vi "Oxford_Data_Recorder.vi"() -> ()   [LabVIEW 2021]
uses:
  <instrlib>/Mercury iXX/Public/Controls/Comms Transport Layer.ctl
  <instrlib>/Mercury iXX/Public/Controls/Serial Settings.ctl
  <instrlib>/Mercury iXX/Public/Controls/ISOBus Address.ctl
  <instrlib>/Mercury iXX/Public/Controls/Mercury Reference.ctl
  <instrlib>/Mercury iXX/Private/Controls/Query Dynamic Reference.ctl
  <instrlib>/Stanford Research 830/Public/Data/Read (All Parameters).vi
  <instrlib>/Keithley 24XX/Public/Data/Read (Single Point).vi
  <instrlib>/Mercury iXX/Public/Libraries/System/Open/Open System.vi
  <instrlib>/Mercury iXX/Public/Libraries/System/Read/Catalogue (Read).vi
  <instrlib>/Mercury iXX/Public/Libraries/Magnet/Configuration/Read/Current to Field Factor (Read).vi
  <instrlib>/Mercury iXX/Public/Libraries/Temperature/Signals/Read/Temperature (Read).vi
  <instrlib>/Mercury iXX/Public/Libraries/Magnet/Signals/Read/Current (Read).vi
  <instrlib>/Mercury iXX/Public/Libraries/Magnet/Signals/Read/Voltage (Read).vi
  <instrlib>/Mercury iXX/Public/Libraries/Magnet/Signals/Read/Persistant Current (Read).vi
  <instrlib>/Keithley 24XX/Keithley 24XX.lvlib
  <instrlib>/Stanford Research 830/Stanford Research 830.lvlib
  <instrlib>/Mercury iXX/Mercury iXX.lvlib
  <instrlib>/Mercury iXX/Public/Libraries/System.lvlib
  <instrlib>/Mercury iXX/Public/Libraries/Magnet.lvlib
  <instrlib>/Mercury iXX/Public/Libraries/Temperature.lvlib
panel:
  in  "ISOBUS address 3":T1=-1 caption="ISOBUS address (-1)"
  in  "ISOBUS address 2":T1=-1 caption="ISOBUS address (-1)"
  in  "Mercury Reference In 2":T2
  in  "Mercury Reference In":T2
  in  "ISOBUS address":T1=-1
  in  "Mag_Ref":T2
  out "Device Details":T5
  in  "Connection Details":T7={"VISA resource name"="", "Comms Layer"=enum."Ethernet TCP/IP", "IP Address"="", "Serial Configuration"={"Baud Rate"=9600, "Parity"=0, "Data Bits"=8, "Stop Bits"=10, "Flow Control"=0}, "ISOBUS address"=-1} {"Serial Configuration"."Flow Control" items=["None", "XON/XOFF", "RTS/CTS", "XON/XOFF & RTS/CTS", "DTR/DSR", "XON/XOFF & DTR/DSR"]; "Serial Configuration"."Stop Bits" items=["1.0"=10, "2.0"=20]; "Serial Configuration"."Data Bits" items=["7"=7, "8"=8]; "Serial Configuration"."Parity" items=["None", "Odd", "Even"]; "Serial Configuration"."Baud Rate" items=["300"=300, "600"=600, "1200"=1200, "2400"=2400, "4800"=4800, "9600"=9600, "19200"=19200]}
  out "Phase-Vg":cluster{dbl[], dbl[]}[](graph)
  out "Leak-Vg":cluster{dbl[], dbl[]}[](graph)
  out "Signal-T":cluster{dbl[], dbl[]}[](graph)
  out "Signal-B":cluster{dbl[], dbl[]}[](graph)
  out "Signal-Vg":cluster{dbl[], dbl[]}[](graph)
  out "Voltage #3":sgl
  out "Leakage Current #3":sgl
  out "X-Value 3":dbl
  out "Theta-Value 3":dbl
  out "R-Value 3":dbl
  in  "Keithley #3 Ramp":bool
  in  "Keith#3 Comp. Lvl":dbl=1e-07
  in  "System #3 Enabled/Disabled":bool
  in  "Keithley #3":refnum<visa-resource-name>
  in  "SR830 #3":refnum<visa-resource-name>="GPIB0::10::INSTR"
  in  "SR830 #3 Input Connection":u16(ring) items=["Single-Ended Voltage", "Differential Voltage", "1 MOhm Current Gain", "100 MOhm Current Gain"]
  in  "SR830 #3\nInput Coupling":u16(ring) items=["AC", "DC"]
  in  "SR830 #3 Input \nShield Grounding":u16(ring) items=["Float", "Ground"]
  in  "SR830 #3 Input\nNotch Filter":u16(ring) items=["None", "Line Notch", "2x Line Notch", "Both Notch Filters"]
  in  "SR830 #3 Trigger Source":u16(ring) items=["Internal", "External"]
  in  "SR830 #3 Internal \nReference Frequency":dbl=17.0
  in  "SR830 #3 Detection Harm. Num.":dbl=1.0
  in  "SR830 #3 Sine \nOutput Amplitude":dbl=1.0
  in  "SR830 #3 Reference Source":u16(ring)=1 items=["External", "Internal"]
  in  "SR830 #3 Manual \nPhase":dbl
  in  "SR830 #3 \nAuto Phase":bool
  in  "SR830 #3 \nTime Constant":u16(ring)=9 items=["10 us", "30 us", "100 us", "300 us", "1 ms", "3 ms", "10 ms", "30 ms", "100 ms", "300 ms", "1 s", "3 s", "10 s", "30 s", "100 s", "300 s", "1 ks", "3 ks", "10 ks", "30 ks"]
  in  "SR830 #3 Low\nPass Filter Slope":u16(ring)=3 items=["6 dB/oct", "12 dB/oct", "18 db/oct", "24 dB/oct"]
  in  "SR830 #3\nSync Filter":bool
  in  "SR830 #3 \nDynamic Reserve":i16(ring)=1 items=["Auto Reserve"=-1, "High Reserve"=0, "Normal"=1, "Low Noise"=2]
  in  "SR830 #3\nSensitivity":i16(ring)=17 items=["Auto Gain"=-1, "2 nV/fA"=0, "5 nV/fA"=1, "10 nV/fA"=2, "20 nV/fA"=3, "50 nV/fA"=4, "100 nV/fA"=5, "200 nV/fA"=6, "500 nV/fA"=7, "1 uV/pA"=8, "2 uV/pA"=9, "5 uV/pA"=10, "10 uV/pA"=11, "20 uV/pA"=12, "50 uV/pA"=13, "100 uV/pA"=14, "200 uV/pA"=15, "500 uV/pA"=16, "1 mV/nA"=17, "2 mV/nA"=18, "5 mV/nA"=19, "10 mV/nA"=20, "20 mV/nA"=21, "50 mV/nA"=22, "100 mV/nA"=23, "200 mV/nA"=24, "500 mV/mA"=25, "1 V/uA"=26]
  in  "Keithley #3 Vg Init. (V)":dbl
  in  "Keithley #3 Vg Max (V)":dbl
  in  "Keithley #3 Vg Min (V)":dbl
  in  "Keithley #3 Vg Step (V)":dbl
  out "Voltage #2":sgl
  out "Leakage Current #2":sgl
  out "X-Value 2":dbl
  out "Theta-Value 2":dbl
  out "R-Value 2":dbl
  in  "Keithley #2 Ramp":bool
  in  "Keith#2 Comp. Lvl":dbl=1e-07
  in  "System #2 Enabled/Disabled":bool
  in  "Keithley #2":refnum<visa-resource-name>
  in  "SR830 #2":refnum<visa-resource-name>="GPIB0::10::INSTR"
  in  "SR830 #2 Input Connection":u16(ring) items=["Single-Ended Voltage", "Differential Voltage", "1 MOhm Current Gain", "100 MOhm Current Gain"]
  in  "SR830 #2\nInput Coupling":u16(ring) items=["AC", "DC"]
  in  "SR830 #2 Input \nShield Grounding":u16(ring) items=["Float", "Ground"]
  in  "SR830 #2 Input\nNotch Filter":u16(ring) items=["None", "Line Notch", "2x Line Notch", "Both Notch Filters"]
  in  "SR830 #2 Trigger Source":u16(ring) items=["Internal", "External"]
  in  "SR830 #2 Internal \nReference Frequency":dbl=17.0
  in  "SR830 #2 Detection Harm. Num.":dbl=1.0
  in  "SR830 #2 Sine \nOutput Amplitude":dbl=1.0
  in  "SR830 #2 Reference Source":u16(ring)=1 items=["External", "Internal"]
  in  "SR830 #2 Manual \nPhase":dbl
  in  "SR830 #2 \nAuto Phase":bool
  in  "SR830 #2 \nTime Constant":u16(ring)=9 items=["10 us", "30 us", "100 us", "300 us", "1 ms", "3 ms", "10 ms", "30 ms", "100 ms", "300 ms", "1 s", "3 s", "10 s", "30 s", "100 s", "300 s", "1 ks", "3 ks", "10 ks", "30 ks"]
  in  "SR830 #2 Low\nPass Filter Slope":u16(ring)=3 items=["6 dB/oct", "12 dB/oct", "18 db/oct", "24 dB/oct"]
  in  "SR830 #2\nSync Filter":bool
  in  "SR830 #2 \nDynamic Reserve":i16(ring)=1 items=["Auto Reserve"=-1, "High Reserve"=0, "Normal"=1, "Low Noise"=2]
  in  "SR830 #2\nSensitivity":i16(ring)=17 items=["Auto Gain"=-1, "2 nV/fA"=0, "5 nV/fA"=1, "10 nV/fA"=2, "20 nV/fA"=3, "50 nV/fA"=4, "100 nV/fA"=5, "200 nV/fA"=6, "500 nV/fA"=7, "1 uV/pA"=8, "2 uV/pA"=9, "5 uV/pA"=10, "10 uV/pA"=11, "20 uV/pA"=12, "50 uV/pA"=13, "100 uV/pA"=14, "200 uV/pA"=15, "500 uV/pA"=16, "1 mV/nA"=17, "2 mV/nA"=18, "5 mV/nA"=19, "10 mV/nA"=20, "20 mV/nA"=21, "50 mV/nA"=22, "100 mV/nA"=23, "200 mV/nA"=24, "500 mV/mA"=25, "1 V/uA"=26]
  in  "Keithley #2 Vg Init. (V)":dbl
  in  "Keithley #2 Vg Max (V)":dbl
  in  "Keithley #2 Vg Min (V)":dbl
  in  "Keithley #2 Vg Step (V)":dbl
  out "Temperature":dbl
  out "Field":dbl
  in  "Remote":bool
  out "Chamber Status":i32(ring) items=["ChamberUnknown"=0, "PurgedAndSealed"=1, "VentedAndSealed"=2, "Sealed"=3, "Purging"=4, "Venting"=5, "PreHiVac"=6, "HighVac"=7, "PumpContinuous"=8, "VentContinuous"=9, "ChamberFailure"=15]
  out "Measuring":bool
  out "R-Value":dbl
  out "Theta-Value":dbl
  out "X-Value":dbl
  out "Leakage Current #1":sgl
  out "Voltage #1":sgl
  in  "Keithley #1 Ramp":bool
  in  "Keith#1 Comp. Lvl":dbl=1e-07
  in  "Keithley #1 Vg Step (V)":dbl
  in  "Keithley #1 Vg Max (V)":dbl
  in  "Keithley #1 Vg Min (V)":dbl
  in  "Keithley #1 Vg Init. (V)":dbl
  in  "Keithley #1":refnum<visa-resource-name>
  in  "SR830 #1\nSensitivity":i16(ring)=17 items=["Auto Gain"=-1, "2 nV/fA"=0, "5 nV/fA"=1, "10 nV/fA"=2, "20 nV/fA"=3, "50 nV/fA"=4, "100 nV/fA"=5, "200 nV/fA"=6, "500 nV/fA"=7, "1 uV/pA"=8, "2 uV/pA"=9, "5 uV/pA"=10, "10 uV/pA"=11, "20 uV/pA"=12, "50 uV/pA"=13, "100 uV/pA"=14, "200 uV/pA"=15, "500 uV/pA"=16, "1 mV/nA"=17, "2 mV/nA"=18, "5 mV/nA"=19, "10 mV/nA"=20, "20 mV/nA"=21, "50 mV/nA"=22, "100 mV/nA"=23, "200 mV/nA"=24, "500 mV/mA"=25, "1 V/uA"=26]
  in  "SR830 #1 \nDynamic Reserve":i16(ring)=1 items=["Auto Reserve"=-1, "High Reserve"=0, "Normal"=1, "Low Noise"=2]
  in  "SR830 #1\nSync Filter":bool
  in  "SR830 #1 Low\nPass Filter Slope":u16(ring)=3 items=["6 dB/oct", "12 dB/oct", "18 db/oct", "24 dB/oct"]
  in  "SR830 #1 \nTime Constant":u16(ring)=8 items=["10 us", "30 us", "100 us", "300 us", "1 ms", "3 ms", "10 ms", "30 ms", "100 ms", "300 ms", "1 s", "3 s", "10 s", "30 s", "100 s", "300 s", "1 ks", "3 ks", "10 ks", "30 ks"]
  in  "SR830 #1 \nAuto Phase":bool
  in  "SR830 #1 Manual \nPhase":dbl
  in  "SR830 #1 Reference Source":u16(ring)=1 items=["External", "Internal"]
  in  "SR830 #1 Sine \nOutput Amplitude":dbl=1.0
  in  "SR830 #1 Detection Harm. Num.":dbl=1.0
  in  "SR830 #1 Internal \nReference Frequency":dbl=17.0
  in  "SR830 #1 Trigger Source":u16(ring) items=["Internal", "External"]
  in  "SR830 #1 Input\nNotch Filter":u16(ring) items=["None", "Line Notch", "2x Line Notch", "Both Notch Filters"]
  in  "SR830 #1 Input \nShield Grounding":u16(ring) items=["Float", "Ground"]
  in  "SR830 #1\nInput Coupling":u16(ring) items=["AC", "DC"]
  in  "SR830 #1 Input Connection":u16(ring) items=["Single-Ended Voltage", "Differential Voltage", "1 MOhm Current Gain", "100 MOhm Current Gain"]
  in  "SR830 #1":refnum<visa-resource-name>="GPIB0::10::INSTR"
  in  "System #1 Enabled/Disabled":bool
  in  "System Reset All?":bool
  in  "program_stop":bool
  out "Actual Save Path":path
  in  "<File Name>.txt (Don't add extension)":string
  in  "Data Save Path:":path=path "C:/Users/Nanonis Tramea/Documents/Data saving/User"
  # "Readout (Recorded)"
  # "Keithley 24XX"
  # "Ramp Settings"
  # "Current Compliance"
  # "SR830"
  # "Input Signal"
  # "Readout (Recorded)"
  # "Source / Reference"
  # "Input Filters & Sens"
  # "Readout (Recorded)"
  # "Keithley 24XX"
  # "Ramp Settings"
  # "Current Compliance"
  # "SR830"
  # "Input Signal"
  # "Readout (Recorded)"
  # "Source / Reference"
  # "Input Filters & Sens"
  # "PPMS"
  # "Readout (Recorded)"
  # "Keithley 24XX"
  # "Ramp Settings"
  # "Current Compliance"
  # "SR830"
  # "Input Signal"
  # "Readout (Recorded)"
  # "Source / Reference"
  # "Input Filters & Sens"
  # "Initialisation:\n--> Reset \n--> Instruments?"
  # "File I/O"
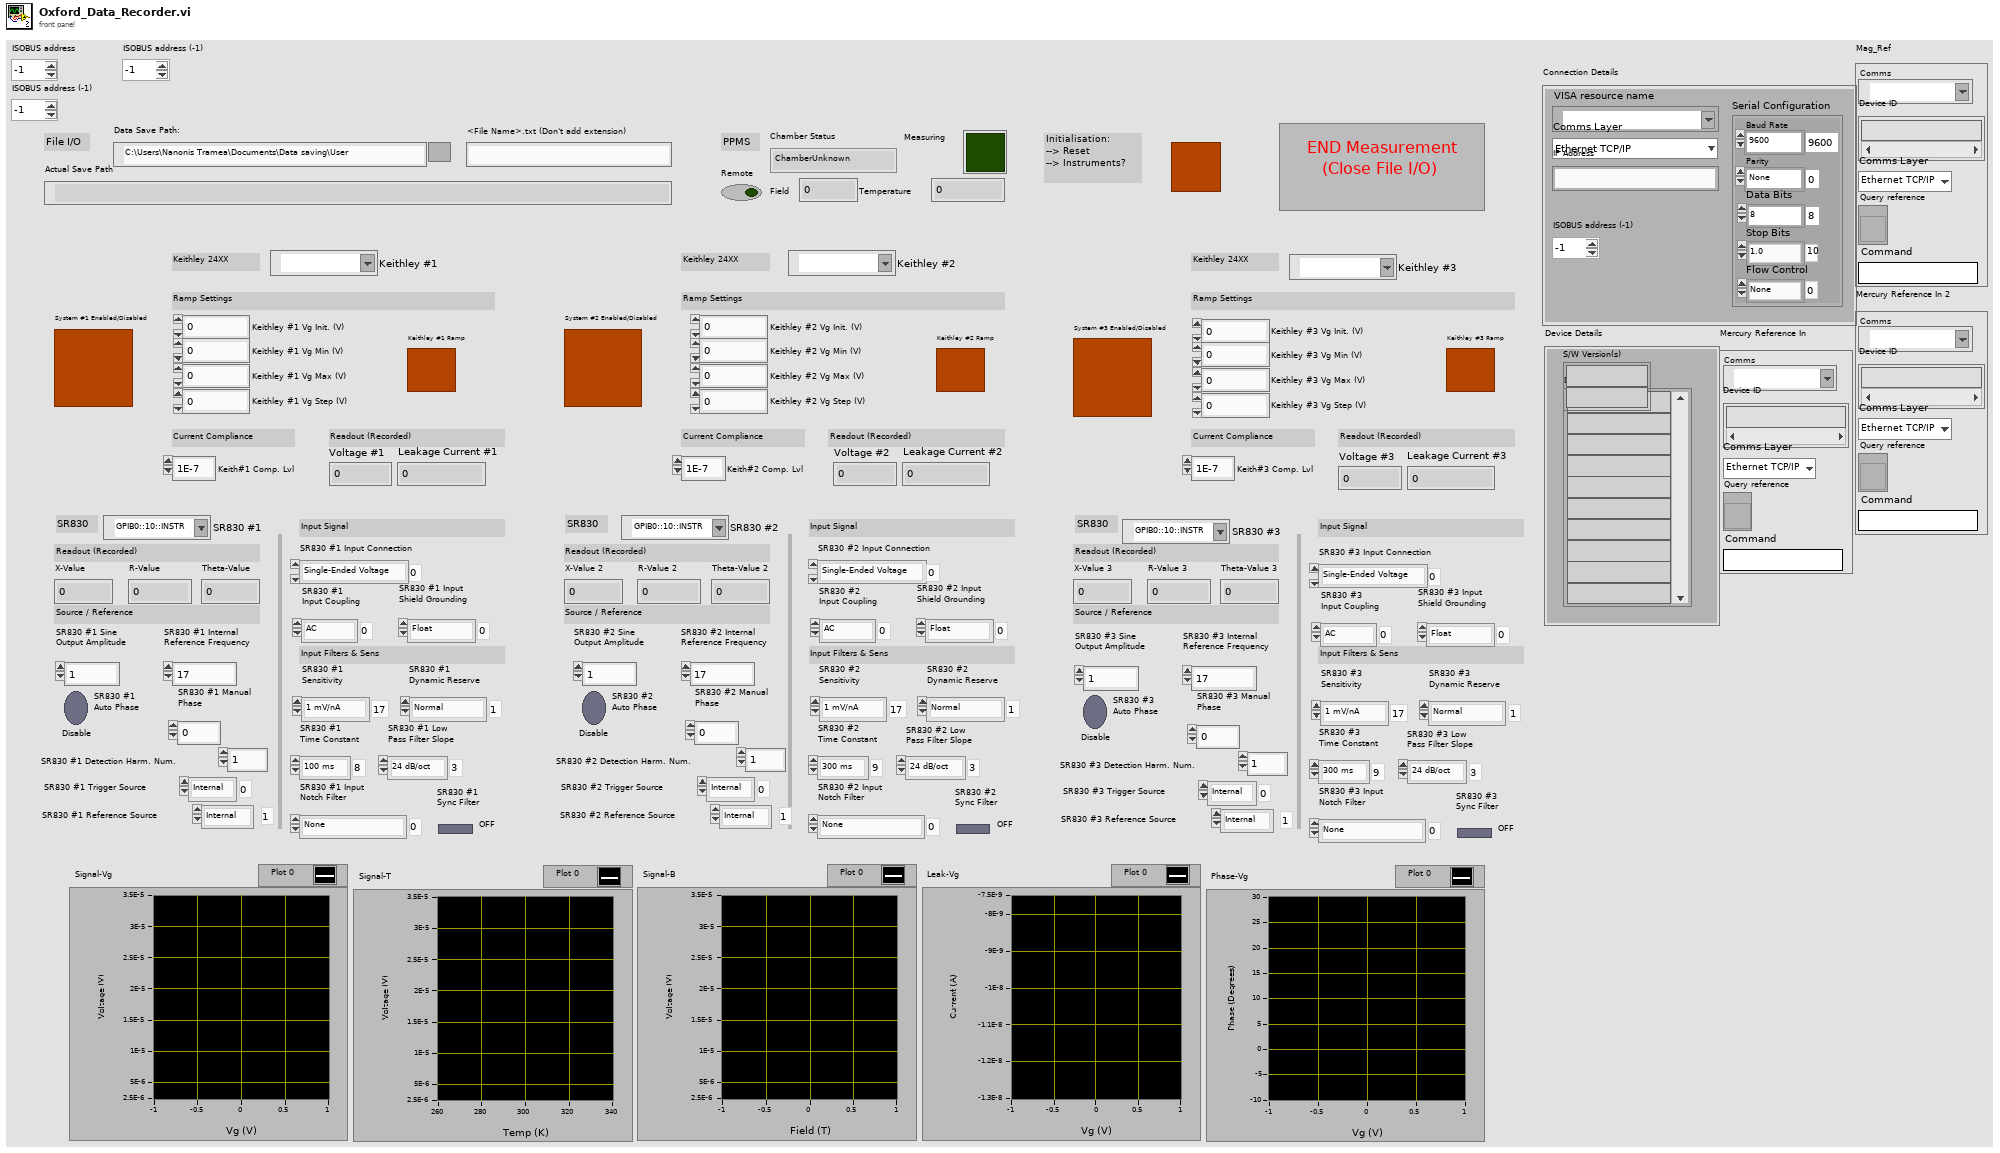
[diagram p1: front panel]
types:
  T1 = typedef "Mercury iXX.lvlib/ISOBus Address.ctl" = i32
  T2 = typedef "Mercury iXX.lvlib/Mercury Reference.ctl" = cluster{"Comms":refnum<visa-resource-name>, "Device ID":string[], "Comms Layer":T3, "Command":string, "Query reference":T4}
  T3 = typedef "Mercury iXX.lvlib/Comms Transport Layer.ctl" = enum16{"Ethernet TCP/IP", "USB", "ISOBus - RS-232", "GPIB"}
  T4 = typedef "Mercury iXX.lvlib/Query Dynamic Reference.ctl" = refnum<vi>
  T5 = cluster{"Devices":string[], "S/W Version(s)":string[]}
  T6 = typedef "Mercury iXX.lvlib/Serial Settings.ctl" = cluster{"Baud Rate":u32, "Parity":u16, "Data Bits":u16, "Stop Bits":u16, "Flow Control":u16}
  T7 = cluster{"VISA resource name":refnum<visa-resource-name>, "Comms Layer":T3, "IP Address":string, "Serial Configuration":T6, "ISOBUS address":T1}
  T8 = enum16{"open", "replace", "create", "open or create", "replace or create", "replace or create with confirmation"}
  T9 = cluster{"System #1 Enabled/Disabled":bool, "System #2 Enabled/Disabled":bool, "System #3 Enabled/Disabled":bool}
  T10 = cluster{"VISA resource name out":refnum<visa-resource-name>, "error out":errorcluster, "VISA resource name out":refnum<visa-resource-name>, "error out":errorcluster, "Keithley #1 Vg Init. (V)":dbl, "Keithley #1 Vg Max (V)":dbl, "Keithley #1 Vg Min (V)":dbl, "Keithley #1 Vg Step (V)":dbl, "Keith#1 Comp. Lvl":dbl}
  T11 = cluster{"Baud Rate":u32, "Parity":u16, "Data Bits":u16, "Stop Bits":u16, "Flow Control":u16}
  T12 = cluster{"VISA resource name out":refnum<visa-resource-name>, "error out":errorcluster, "VISA resource name out":refnum<visa-resource-name>, "error out":errorcluster, "Keithley #2 Vg Init. (V)":dbl, "Keithley #2 Vg Max (V)":dbl, "Keithley #2 Vg Min (V)":dbl, "Keithley #2 Vg Step (V)":dbl, "Keith#2 Comp. Lvl":dbl}
  T13 = cluster{"VISA resource name out":refnum<visa-resource-name>, "error out":errorcluster, "VISA resource name out":refnum<visa-resource-name>, "error out":errorcluster, "Keithley #3 Vg Init. (V)":dbl, "Keithley #3 Vg Max (V)":dbl, "Keithley #3 Vg Min (V)":dbl, "Keithley #3 Vg Step (V)":dbl, "Keith#3 Comp. Lvl":dbl}
  T14 = cluster{"array":dbl[][], "array":dbl[][], "array":dbl[][], "array":dbl[][]}
  T15 = cluster{"Voltage":sgl, "Current":sgl, "X-Value":dbl, "R-Value":dbl, "Theta-Value":dbl}
  T16 = enum8{"Enabled", "Disabled", "Disabled and Grayed Out"}
  T17 = cluster{"X-Value":dbl, "Y-Value":dbl, "R-Value":dbl, "Theta-Value":dbl, "Aux In 1 Value":dbl, "Aux In 2 Value":dbl, "Aux In 3 Value":dbl, "Aux In 4 Value":dbl, "Reference Frequency":dbl, "Channel 1 Display":dbl, "Channel 2 Display":dbl}
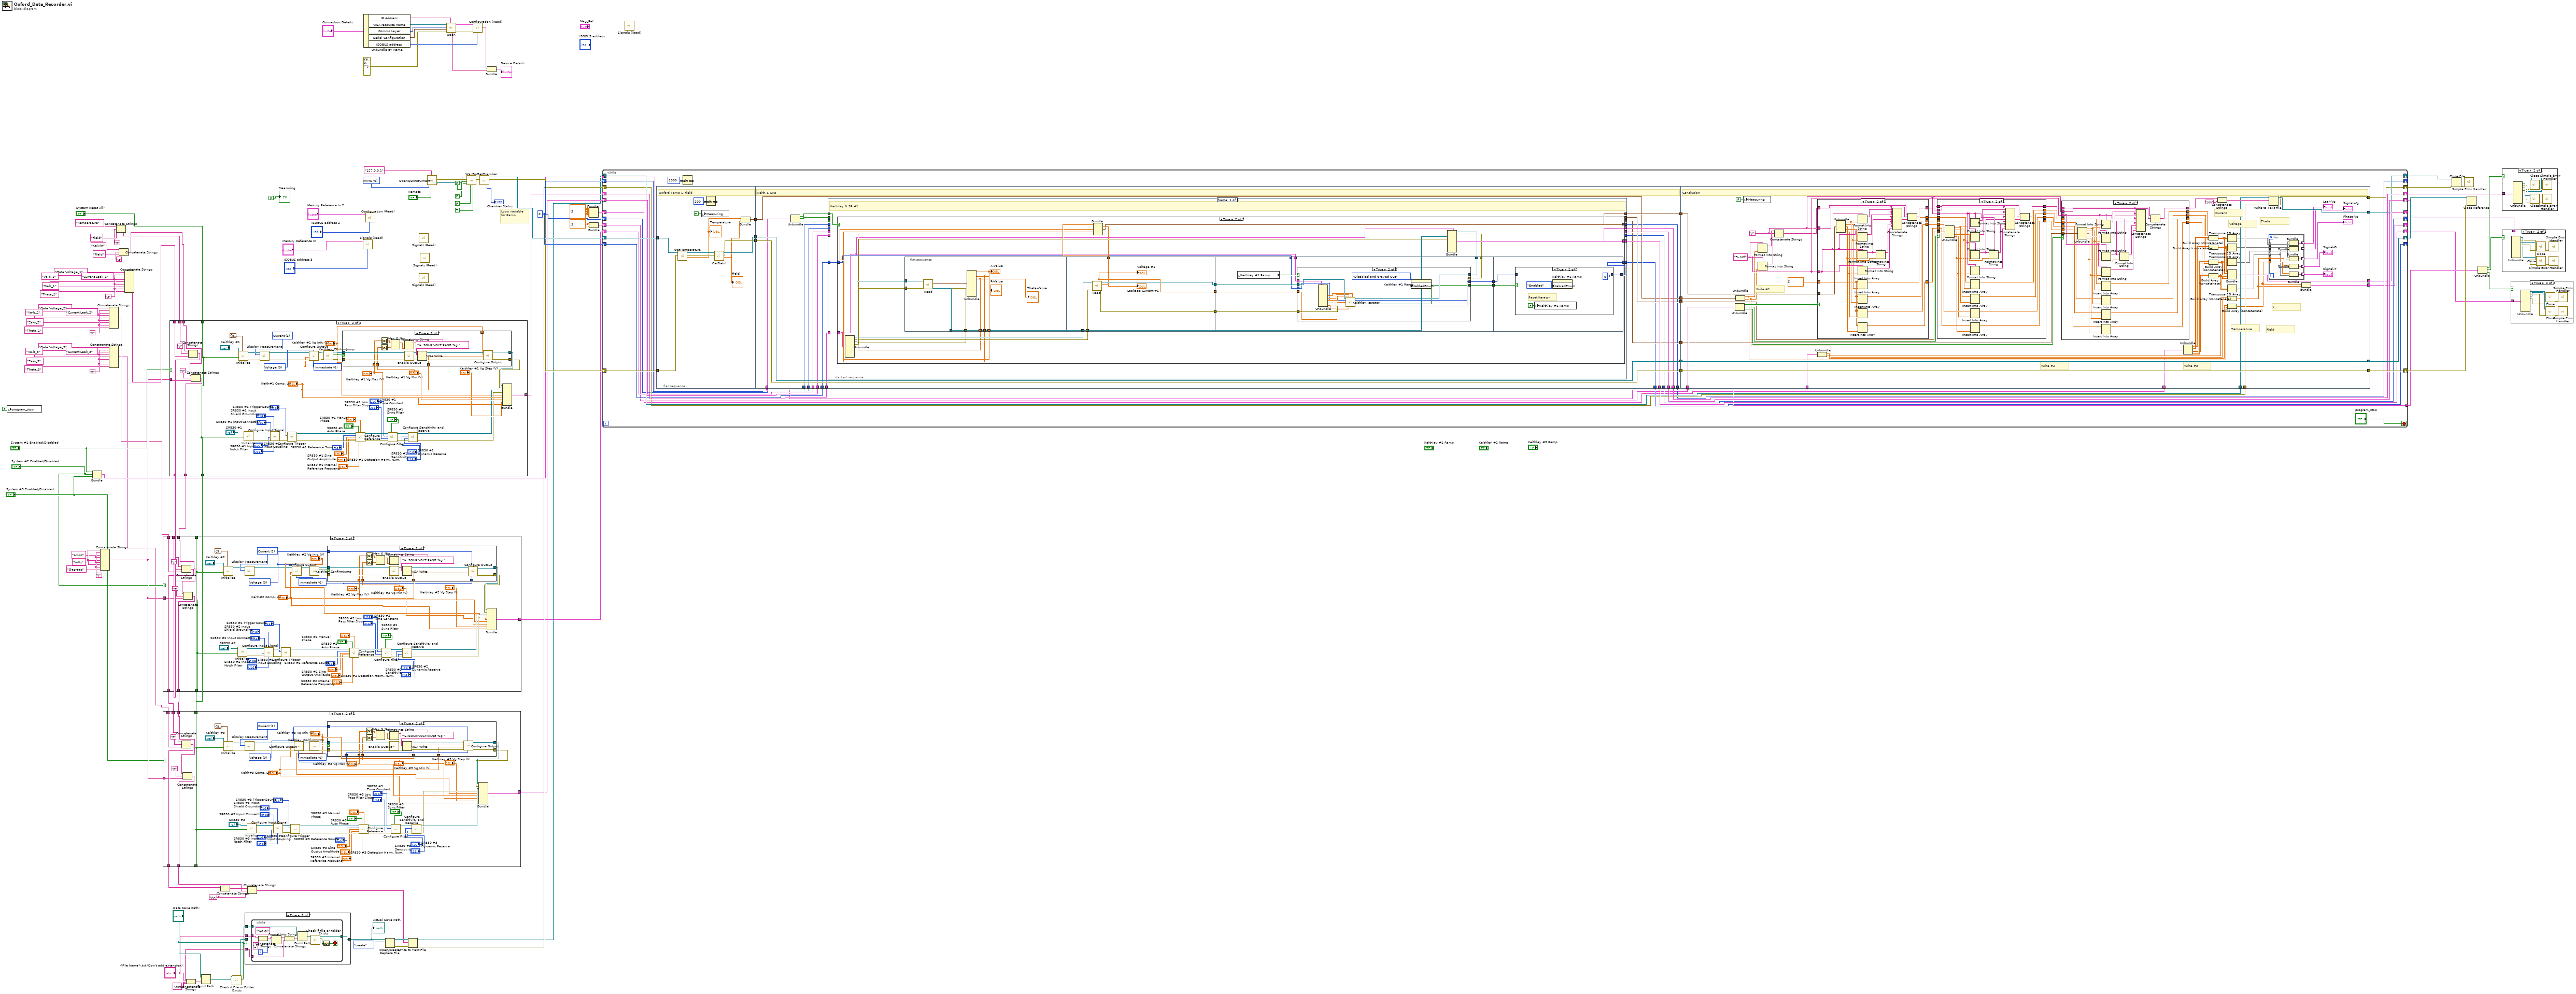
[diagram p0: block diagram]
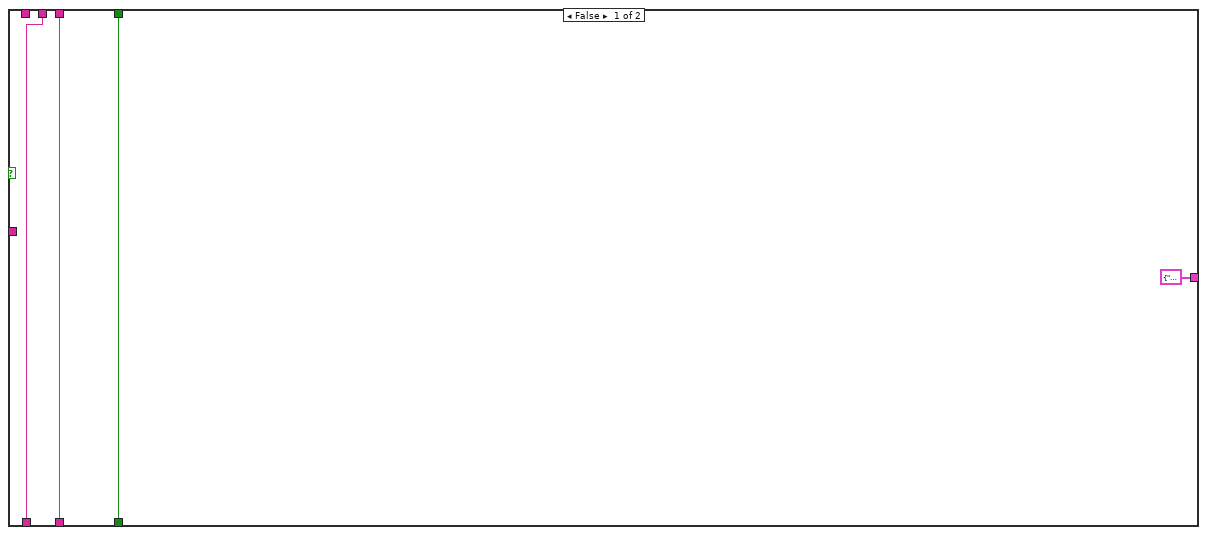
[diagram p5: hidden frame]
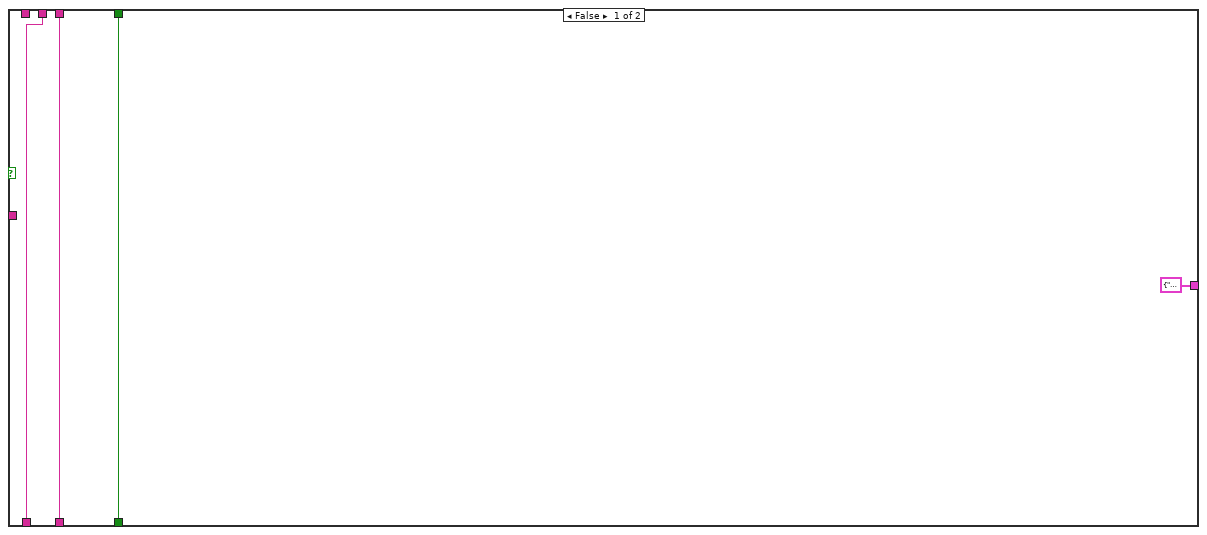
[diagram p7: hidden frame]
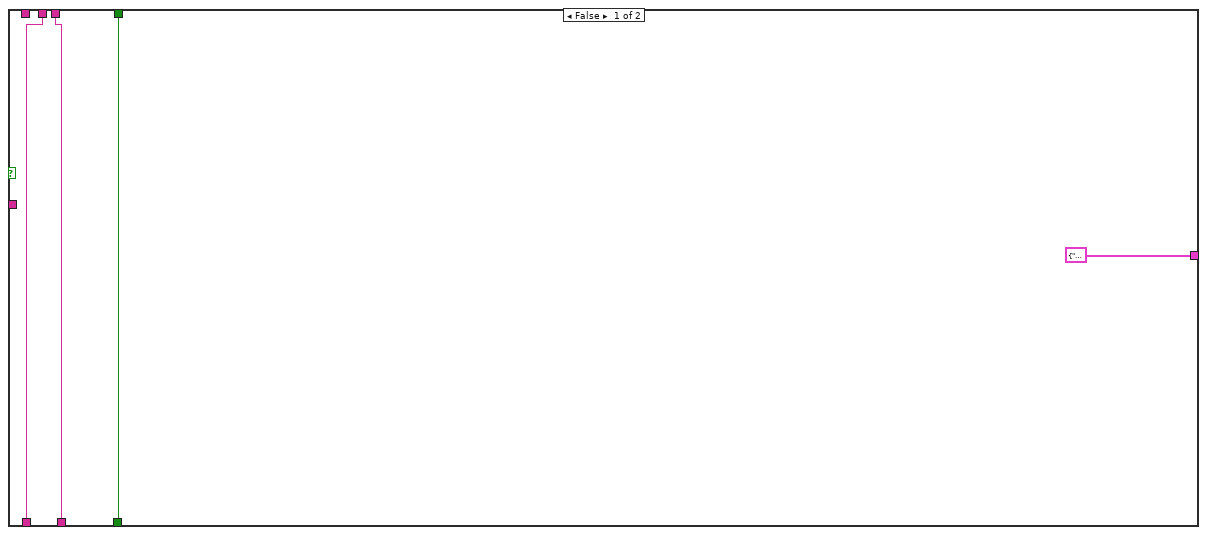
[diagram p9: hidden frame]
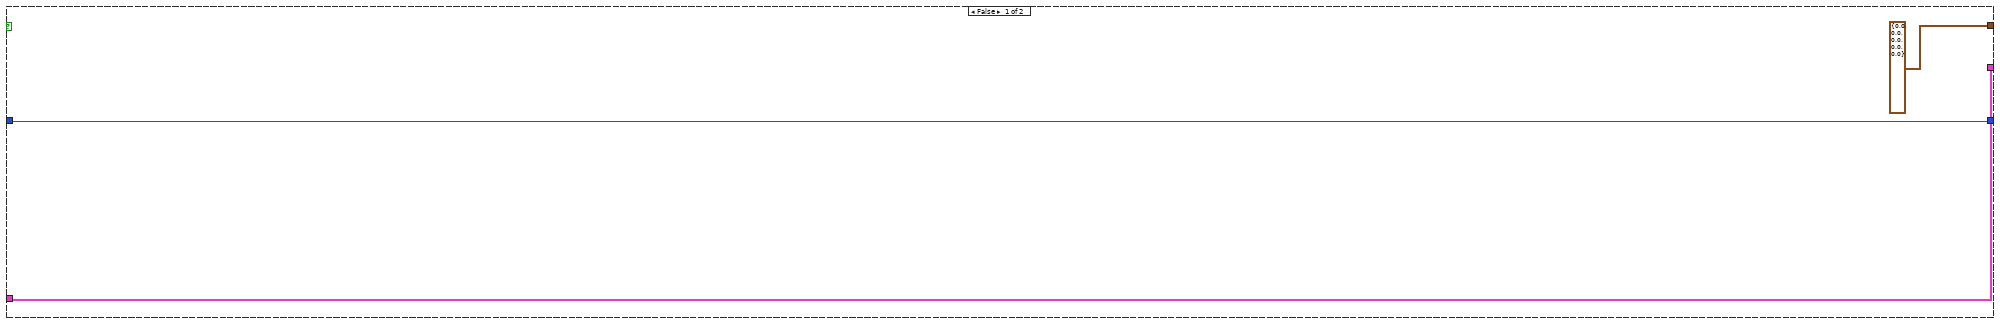
[diagram p12: hidden frame]
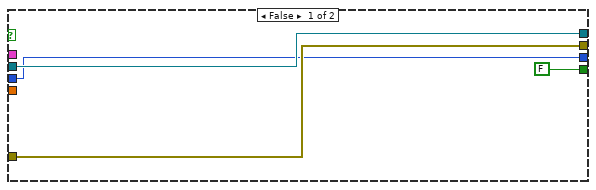
[diagram p13: hidden frame]
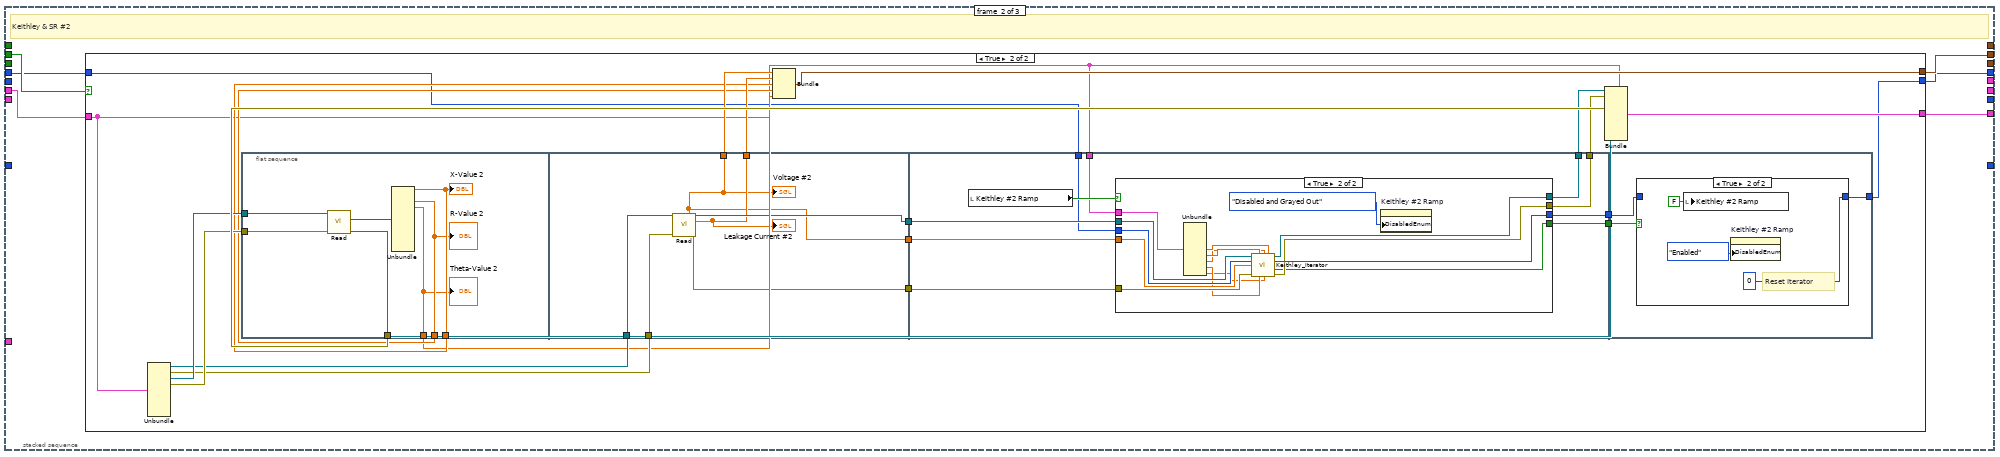
[diagram p15: hidden frame]
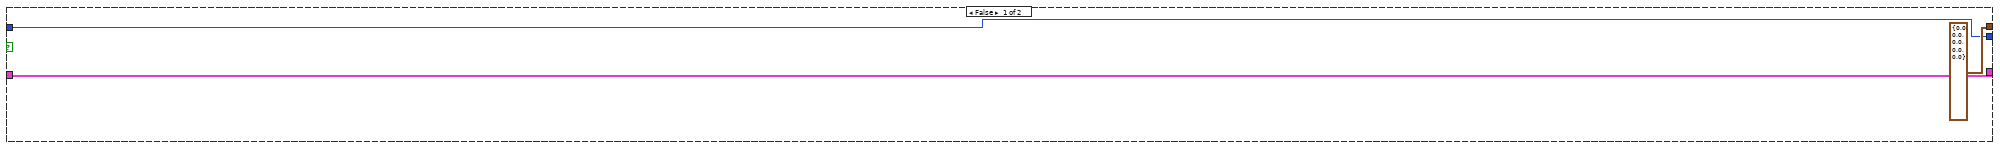
[diagram p16: hidden frame]
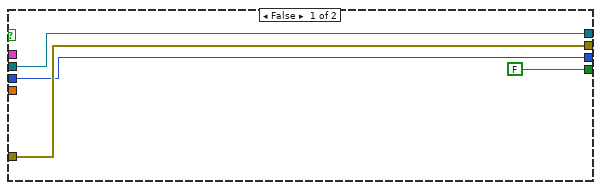
[diagram p17: hidden frame]
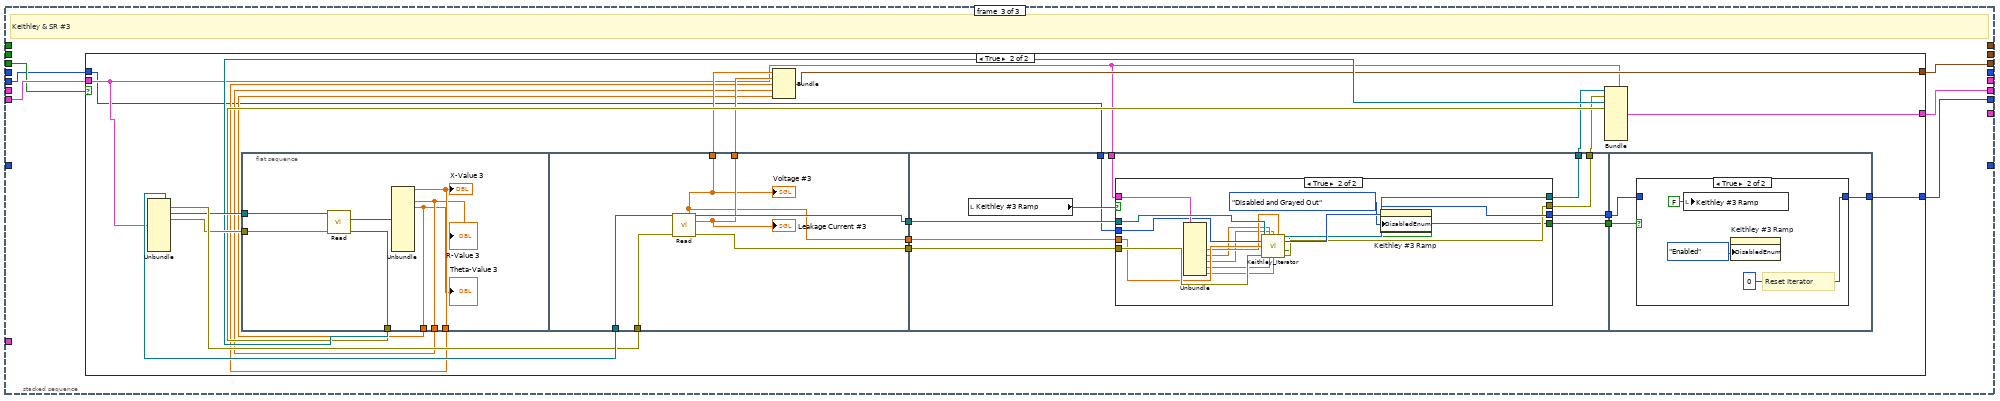
[diagram p19: hidden frame]
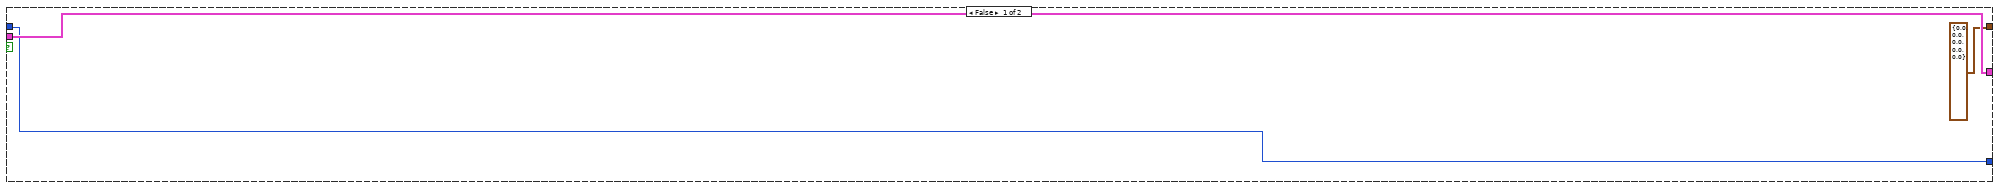
[diagram p20: hidden frame]
diagram:
  w26 = "\t"
  w32 = "\t"
  w42 = dbl[][] [] ("array")
  w44 = dbl[] [] ("array")
  w66 = 0
  w81 = "\t"
  w18 = "Volts" ("string")
  w70 = "\r\n"
  w90 = "\t"
  w95 = 0 items=["PPMS", "VersaLab", "DynaCool", "SVSM"] ("Instrument Type")
  w98 = ".txt"
  # "Loop variable \nfor Ramp"
  n1 = local write "program_stop"(FALSE ("program_stop")) -> ()
  n2 = Bundle("System #1 Enabled/Disabled"="System #1 Enabled/Disabled", "System #2 Enabled/Disabled"="System #2 Enabled/Disabled", "System #3 Enabled/Disabled"="System #3 Enabled/Disabled") -> (w51:T9)  [unwired: 1 in]
  n3 = Concatenate Strings(w18, w81, "Amps" ("string"), w81, w18, w81, w18, w81, "Degrees" ("string")) -> (w73:string)
  n4 = Concatenate Strings("Gate Voltage_2" ("string"), w32, "Current Leak_2" ("string"), w32, "Va-b_2" ("string"), w32, "Za-b_2" ("string"), w32, "Theta_2" ("string")) -> (w21:string)
  n5 = Concatenate Strings("Gate Voltage_3" ("string"), w26, "Current Leak_3" ("string"), w26, "Va-b_3" ("string"), w26, "Za-b_3" ("string"), w26, "Theta_3" ("string")) -> (w20:string)
  n6 = Concatenate Strings("Temperature" ("string"), "\t", "Field" ("string")) -> (w89:string)
  n7 = Concatenate Strings("Kelvin" ("string"), "\t", "Field" ("string")) -> (w76:string)
  n8 = Concatenate Strings("Gate Voltage_1" ("string"), w90, "Current Leak_1" ("string"), w90, "Va-b_1" ("string"), w90, "Za-b_1" ("string"), w90, "Theta_1" ("string")) -> (w84:string)
  n9 = case shown="True" "System #1 Enabled/Disabled" {
    tunnel: w84 -> [_ w179]
    tunnel: w89 -> [w119 w177]
    tunnel: [w119 w176] -> w87
    tunnel: "System Reset All?" -> [w118 w134]
    tunnel: [w118 w134] -> w86
    tunnel: w76 -> [w117 w132]
    tunnel: [w117 w131] -> w75
    tunnel: w73 -> [_ w130]
    tunnel: [T10 {"VISA resource name out"="", "error out"={"status"=FALSE, "code"=0, "source"=""}, "VISA resource name out"="", "error out"={"status"=FALSE, "code"=0, "source"=""}, "Keithley #1 Vg Init. (V)"=0.0, "Keithley #1 Vg Max (V)"=0.0, "Keithley #1 Vg Min (V)"=0.0, "Keithley #1 Vg Step (V)"=0.0, "Keith#1 Comp. Lvl"=0.0} w122] -> w57
    frame False {
    }
    frame True {
      w140 = u16 0 items=["Immediate", "Triggered"] ("Output Type  (0: Immediate)")
      w139 = u16 0 items=["Voltage", "Current"] ("Source Mode  (0: Voltage)")
      w174 = u16 1 items=["Voltage", "Current", "Resistance"] ("Displayed Measurement (0: Voltage)")
      n10 = Concatenate Strings(w177, "\t", w179) -> (w176:string)
      n11 = Concatenate Strings(w132, "\t", w130) -> (w131:string)
      n12 = call <instrlib>:"Initialize.vi"("Serial Configuration"=T11 {"Baud Rate"=9600, "Parity"=0, "Data Bits"=8, "Stop Bits"=10, "Flow Control"=0}, "Reset (True)"=w134, "VISA resource name"="Keithley #1") -> ("error out"=w172:errorcluster, "VISA resource name out"=w173:refnum<visa-resource-name>)  [unwired: 7 in]
      n13 = call <instrlib>:"Initialize.vi"("Reset (True)"=w134, "VISA resource name"="SR830 #1") -> ("error out"=w166:errorcluster, "VISA resource name out"=w167:refnum<visa-resource-name>)  [unwired: 8 in]
      n14 = call <instrlib>:"Display Measurement.vi"("error in (no error)"=w172, "Displayed Measurement (0: Voltage)"=w174, "VISA resource name"=w173) -> ("error out"=w137:errorcluster, "VISA resource name out"=w138:refnum<visa-resource-name>)  [unwired: 7 in]
      n15 = call <instrlib>:"Configure Input Signal.vi"("Input Notch Filter (0: None)"="SR830 #1 Input\nNotch Filter", "Input Shield Grounding (0: Float)"="SR830 #1 Input \nShield Grounding", "error in (no error)"=w166, "Input Coupling (0: AC)"="SR830 #1\nInput Coupling", "Input Connection (0: Single-Ended Voltage)"="SR830 #1 Input Connection", "VISA resource name"=w167) -> ("error out"=w164:errorcluster, "VISA resource name out"=w165:refnum<visa-resource-name>)  [unwired: 4 in]
      n16 = call <instrlib>:"Configure Trigger.vi"("error in (no error)"=w164, "Trigger Source (0: Internal)"="SR830 #1 Trigger Source", "VISA resource name"=w165) -> ("error out"=w162:errorcluster, "VISA resource name out"=w163:refnum<visa-resource-name>)  [unwired: 7 in]
      n17 = call <instrlib>:"Configure Output.vi"("Output Type  (0: Immediate)"=w140, "Source Mode  (0: Voltage)"=w139, "error in (no error)"=w137, "Compliance  Level (0.1)"="Keith#1 Comp. Lvl", "VISA resource name"=w138) -> ("error out"=w135:errorcluster, "VISA resource name out"=w136:refnum<visa-resource-name>)  [unwired: 5 in]
      n18 = call "Keithley_ConfirmJump.vi"("VISA resource name in"=w136, "error in"=w135, "Gate Voltage\nInitial (V)"="Keithley #1 Vg Init. (V)") -> ("VISA resource name out"=w142:refnum<visa-resource-name>, "Voltage OK?"=w143:bool, "error out"=w141:errorcluster)  [unwired: 4 in, 1 out]
      n19 = case shown="True" w143 {
        tunnel: w142 -> [w181 w191]
        tunnel: w141 -> [w180 w190]
        tunnel: [w181 w184] -> w126
        tunnel: [w180 w185] -> w125
        tunnel: "Keithley #1 Vg Max (V)" -> [_ w189]
        tunnel: "Keithley #1 Vg Min (V)" -> [_ w188]
        tunnel: "Keithley #1 Vg Init. (V)" -> [_ w183]
        tunnel: "Keith#1 Comp. Lvl" -> [_ w182]
        frame False {
        }
        frame True {
          n20 = Absolute Value(x=w189) -> (abs(x)=w193:dbl)
          n21 = Absolute Value(x=w188) -> (abs(x)=w194:dbl)
          n22 = Max & Min(x=w193, y=w194) -> (max(x,y)=w198:dbl)  [unwired: 1 out]
          n23 = Format Into String(format string="%.;SOUR:VOLT:RANG %g ", w198) -> (resulting string=w197:string)  [unwired: 2 in, 1 out]
          n24 = call <instrlib>:"Enable Output.vi"("error in (no error)"=w190, "VISA resource name"=w191) -> ("error out"=w195:errorcluster, "VISA resource name out"=w196:refnum<visa-resource-name>)  [unwired: 8 in]
          n25 = VISA Write(VISA resource name=w196, write buffer=w197, error in (no error)=w195) -> (VISA resource name out=w187:refnum<visa-resource-name>, error out=w186:errorcluster)  [unwired: 1 out]
          n26 = call <instrlib>:"Configure Output.vi"("error in (no error)"=w186, "Compliance  Level (0.1)"=w182, "Output Level (0)"=w183, "VISA resource name"=w187) -> ("error out"=w185:errorcluster, "VISA resource name out"=w184:refnum<visa-resource-name>)  [unwired: 6 in]
        }
      }
      n27 = call <instrlib>:"Configure Reference.vi"("VISA resource name"=w163, "Auto Phase (T: Enabled)"="SR830 #1 \nAuto Phase", "Manual Phase (0 Degree)"="SR830 #1 Manual \nPhase", "Reference Source (1: Internal)"="SR830 #1 Reference Source", "Sine Output Amplitude (1 V)"="SR830 #1 Sine \nOutput Amplitude", "Detection Harmonic Number (1)"="SR830 #1 Detection Harm. Num.", "error in (no error)"=w162, "Internal Reference Frequency (1000 Hz)"="SR830 #1 Internal \nReference Frequency") -> ("VISA resource name out"=w160:refnum<visa-resource-name>, "error out"=w161:errorcluster)  [unwired: 6 in]
      n28 = call <instrlib>:"Configure Filter.vi"("Enable Sync Filter (F: Disable)"="SR830 #1\nSync Filter", "error in (no error)"=w161, "Low Pass Filter Slope (1: 12dB/oct)"="SR830 #1 Low\nPass Filter Slope", "Time Constant (8: 100ms)"="SR830 #1 \nTime Constant", "VISA resource name"=w160) -> ("error out"=w146:errorcluster, "VISA resource name out"=w147:refnum<visa-resource-name>)  [unwired: 5 in]
      n29 = call <instrlib>:"Configure Sensitivity and Reserve.vi"("error in (no error)"=w146, "Sensitivity (-1: Auto gain)"="SR830 #1\nSensitivity", "Dynamic Reserve (-1: Auto Reserve)"="SR830 #1 \nDynamic Reserve", "VISA resource name"=w147) -> ("error out"=w123:errorcluster, "VISA resource name out"=w124:refnum<visa-resource-name>)  [unwired: 6 in]
      n30 = Bundle("VISA resource name out"=w126, "error out"=w125, "VISA resource name out"=w124, "error out"=w123, "Keithley #1 Vg Init. (V)"="Keithley #1 Vg Init. (V)", "Keithley #1 Vg Max (V)"="Keithley #1 Vg Max (V)", "Keithley #1 Vg Min (V)"="Keithley #1 Vg Min (V)", "Keithley #1 Vg Step (V)"="Keithley #1 Vg Step (V)", "Keith#1 Comp. Lvl"="Keith#1 Comp. Lvl") -> (w122:T10)  [unwired: 1 in]
    }
  }
  n31 = case shown="True" "System #2 Enabled/Disabled" {
    tunnel: w21 -> [_ w262]
    tunnel: w87 -> [w202 w260]
    tunnel: [w202 w259] -> w85
    tunnel: w86 -> [w201 w223]
    tunnel: [w201 w223] -> w83
    tunnel: w75 -> [w200 w221]
    tunnel: [w200 w220] -> w74
    tunnel: w73 -> [_ w219]
    tunnel: [T12 {"VISA resource name out"="", "error out"={"status"=FALSE, "code"=0, "source"=""}, "VISA resource name out"="", "error out"={"status"=FALSE, "code"=0, "source"=""}, "Keithley #2 Vg Init. (V)"=0.0, "Keithley #2 Vg Max (V)"=0.0, "Keithley #2 Vg Min (V)"=0.0, "Keithley #2 Vg Step (V)"=0.0, "Keith#2 Comp. Lvl"=0.0} w210] -> w56
    frame False {
    }
    frame True {
      w203 = u16 0 items=["Immediate", "Triggered"] ("Output Type  (0: Immediate)")
      w204 = u16 0 items=["Voltage", "Current"] ("Source Mode  (0: Voltage)")
      w257 = u16 1 items=["Voltage", "Current", "Resistance"] ("Displayed Measurement (0: Voltage)")
      n32 = Concatenate Strings(w260, "\t", w262) -> (w259:string)
      n33 = Concatenate Strings(w221, "\t", w219) -> (w220:string)
      n34 = call <instrlib>:"Initialize.vi"("Serial Configuration"=T11 {"Baud Rate"=9600, "Parity"=0, "Data Bits"=8, "Stop Bits"=10, "Flow Control"=0}, "Reset (True)"=w223, "VISA resource name"="Keithley #2") -> ("error out"=w255:errorcluster, "VISA resource name out"=w256:refnum<visa-resource-name>)  [unwired: 7 in]
      n35 = call <instrlib>:"Initialize.vi"("Reset (True)"=w223, "VISA resource name"="SR830 #2") -> ("error out"=w249:errorcluster, "VISA resource name out"=w250:refnum<visa-resource-name>)  [unwired: 8 in]
      n36 = call <instrlib>:"Display Measurement.vi"("error in (no error)"=w255, "Displayed Measurement (0: Voltage)"=w257, "VISA resource name"=w256) -> ("error out"=w208:errorcluster, "VISA resource name out"=w209:refnum<visa-resource-name>)  [unwired: 7 in]
      n37 = call <instrlib>:"Configure Input Signal.vi"("Input Notch Filter (0: None)"="SR830 #2 Input\nNotch Filter", "Input Shield Grounding (0: Float)"="SR830 #2 Input \nShield Grounding", "error in (no error)"=w249, "Input Coupling (0: AC)"="SR830 #2\nInput Coupling", "Input Connection (0: Single-Ended Voltage)"="SR830 #2 Input Connection", "VISA resource name"=w250) -> ("error out"=w247:errorcluster, "VISA resource name out"=w248:refnum<visa-resource-name>)  [unwired: 4 in]
      n38 = call <instrlib>:"Configure Trigger.vi"("error in (no error)"=w247, "Trigger Source (0: Internal)"="SR830 #2 Trigger Source", "VISA resource name"=w248) -> ("error out"=w245:errorcluster, "VISA resource name out"=w246:refnum<visa-resource-name>)  [unwired: 7 in]
      n39 = call <instrlib>:"Configure Output.vi"("Output Type  (0: Immediate)"=w203, "Source Mode  (0: Voltage)"=w204, "error in (no error)"=w208, "Compliance  Level (0.1)"="Keith#2 Comp. Lvl", "VISA resource name"=w209) -> ("error out"=w206:errorcluster, "VISA resource name out"=w205:refnum<visa-resource-name>)  [unwired: 5 in]
      n40 = call "Keithley_ConfirmJump.vi"("VISA resource name in"=w205, "error in"=w206, "Gate Voltage\nInitial (V)"="Keithley #2 Vg Init. (V)") -> ("VISA resource name out"=w225:refnum<visa-resource-name>, "Voltage OK?"=w226:bool, "error out"=w224:errorcluster)  [unwired: 4 in, 1 out]
      n41 = case shown="True" w226 {
        tunnel: w225 -> [w264 w275]
        tunnel: w224 -> [w263 w274]
        tunnel: [w264 w266] -> w218
        tunnel: [w263 w265] -> w217
        tunnel: "Keithley #2 Vg Max (V)" -> [_ w273]
        tunnel: "Keithley #2 Vg Min (V)" -> [_ w272]
        tunnel: w203 -> [_ w271]
        tunnel: w204 -> [_ w270]
        tunnel: "Keith#2 Comp. Lvl" -> [_ w269]
        frame False {
        }
        frame True {
          n42 = Absolute Value(x=w273) -> (abs(x)=w277:dbl)
          n43 = Absolute Value(x=w272) -> (abs(x)=w278:dbl)
          n44 = Max & Min(x=w277, y=w278) -> (max(x,y)=w282:dbl)  [unwired: 1 out]
          n45 = Format Into String(format string="%.;SOUR:VOLT:RANG %g ", w282) -> (resulting string=w281:string)  [unwired: 2 in, 1 out]
          n46 = call <instrlib>:"Enable Output.vi"("error in (no error)"=w274, "VISA resource name"=w275) -> ("error out"=w279:errorcluster, "VISA resource name out"=w280:refnum<visa-resource-name>)  [unwired: 8 in]
          n47 = VISA Write(VISA resource name=w280, write buffer=w281, error in (no error)=w279) -> (VISA resource name out=w268:refnum<visa-resource-name>, error out=w267:errorcluster)  [unwired: 1 out]
          n48 = call <instrlib>:"Configure Output.vi"("Output Type  (0: Immediate)"=w271, "Source Mode  (0: Voltage)"=w270, "error in (no error)"=w267, "Compliance  Level (0.1)"=w269, "VISA resource name"=w268) -> ("error out"=w265:errorcluster, "VISA resource name out"=w266:refnum<visa-resource-name>)  [unwired: 5 in]
        }
      }
      n49 = call <instrlib>:"Configure Reference.vi"("VISA resource name"=w246, "Auto Phase (T: Enabled)"="SR830 #2 \nAuto Phase", "Manual Phase (0 Degree)"="SR830 #2 Manual \nPhase", "Reference Source (1: Internal)"="SR830 #2 Reference Source", "Sine Output Amplitude (1 V)"="SR830 #2 Sine \nOutput Amplitude", "Detection Harmonic Number (1)"="SR830 #2 Detection Harm. Num.", "error in (no error)"=w245, "Internal Reference Frequency (1000 Hz)"="SR830 #2 Internal \nReference Frequency") -> ("VISA resource name out"=w243:refnum<visa-resource-name>, "error out"=w244:errorcluster)  [unwired: 6 in]
      n50 = call <instrlib>:"Configure Filter.vi"("Enable Sync Filter (F: Disable)"="SR830 #2\nSync Filter", "error in (no error)"=w244, "Low Pass Filter Slope (1: 12dB/oct)"="SR830 #2 Low\nPass Filter Slope", "Time Constant (8: 100ms)"="SR830 #2 \nTime Constant", "VISA resource name"=w243) -> ("error out"=w229:errorcluster, "VISA resource name out"=w230:refnum<visa-resource-name>)  [unwired: 5 in]
      n51 = call <instrlib>:"Configure Sensitivity and Reserve.vi"("error in (no error)"=w229, "Sensitivity (-1: Auto gain)"="SR830 #2\nSensitivity", "Dynamic Reserve (-1: Auto Reserve)"="SR830 #2 \nDynamic Reserve", "VISA resource name"=w230) -> ("error out"=w215:errorcluster, "VISA resource name out"=w216:refnum<visa-resource-name>)  [unwired: 6 in]
      n52 = Bundle("VISA resource name out"=w218, "error out"=w217, "VISA resource name out"=w216, "error out"=w215, "Keithley #2 Vg Init. (V)"="Keithley #2 Vg Init. (V)", "Keithley #2 Vg Max (V)"="Keithley #2 Vg Max (V)", "Keithley #2 Vg Min (V)"="Keithley #2 Vg Min (V)", "Keithley #2 Vg Step (V)"="Keithley #2 Vg Step (V)", "Keith#2 Comp. Lvl"="Keith#2 Comp. Lvl") -> (w210:T12)  [unwired: 1 in]
    }
  }
  n53 = case shown="True" "System #3 Enabled/Disabled" {
    tunnel: w20 -> [_ w346]
    tunnel: w85 -> [w286 w344]
    tunnel: [w286 w343] -> w82
    tunnel: w83 -> [w285 w303]
    tunnel: [w285 w303] -> _
    tunnel: w74 -> [w284 w301]
    tunnel: w73 -> [_ w300]
    tunnel: [w284 w299] -> w68
    tunnel: [T13 {"VISA resource name out"="", "error out"={"status"=FALSE, "code"=0, "source"=""}, "VISA resource name out"="", "error out"={"status"=FALSE, "code"=0, "source"=""}, "Keithley #3 Vg Init. (V)"=0.0, "Keithley #3 Vg Max (V)"=0.0, "Keithley #3 Vg Min (V)"=0.0, "Keithley #3 Vg Step (V)"=0.0, "Keith#3 Comp. Lvl"=0.0} w291] -> w55
    frame False {
    }
    frame True {
      w289 = u16 0 items=["Immediate", "Triggered"] ("Output Type  (0: Immediate)")
      w290 = u16 0 items=["Voltage", "Current"] ("Source Mode  (0: Voltage)")
      w341 = u16 1 items=["Voltage", "Current", "Resistance"] ("Displayed Measurement (0: Voltage)")
      n54 = Concatenate Strings(w344, "\t", w346) -> (w343:string)
      n55 = Concatenate Strings(w301, "\t", w300) -> (w299:string)
      n56 = call <instrlib>:"Initialize.vi"("Serial Configuration"=T11 {"Baud Rate"=9600, "Parity"=0, "Data Bits"=8, "Stop Bits"=10, "Flow Control"=0}, "Reset (True)"=w303, "VISA resource name"="Keithley #3") -> ("error out"=w339:errorcluster, "VISA resource name out"=w340:refnum<visa-resource-name>)  [unwired: 7 in]
      n57 = call <instrlib>:"Display Measurement.vi"("error in (no error)"=w339, "Displayed Measurement (0: Voltage)"=w341, "VISA resource name"=w340) -> ("error out"=w306:errorcluster, "VISA resource name out"=w307:refnum<visa-resource-name>)  [unwired: 7 in]
      n58 = call <instrlib>:"Initialize.vi"("Reset (True)"=w303, "VISA resource name"="SR830 #3") -> ("error out"=w333:errorcluster, "VISA resource name out"=w334:refnum<visa-resource-name>)  [unwired: 8 in]
      n59 = call <instrlib>:"Configure Input Signal.vi"("Input Notch Filter (0: None)"="SR830 #3 Input\nNotch Filter", "Input Shield Grounding (0: Float)"="SR830 #3 Input \nShield Grounding", "error in (no error)"=w333, "Input Coupling (0: AC)"="SR830 #3\nInput Coupling", "Input Connection (0: Single-Ended Voltage)"="SR830 #3 Input Connection", "VISA resource name"=w334) -> ("error out"=w331:errorcluster, "VISA resource name out"=w332:refnum<visa-resource-name>)  [unwired: 4 in]
      n60 = call <instrlib>:"Configure Trigger.vi"("error in (no error)"=w331, "Trigger Source (0: Internal)"="SR830 #3 Trigger Source", "VISA resource name"=w332) -> ("error out"=w329:errorcluster, "VISA resource name out"=w330:refnum<visa-resource-name>)  [unwired: 7 in]
      n61 = call <instrlib>:"Configure Output.vi"("Output Type  (0: Immediate)"=w289, "Source Mode  (0: Voltage)"=w290, "error in (no error)"=w306, "Compliance  Level (0.1)"="Keith#3 Comp. Lvl", "VISA resource name"=w307) -> ("error out"=w304:errorcluster, "VISA resource name out"=w305:refnum<visa-resource-name>)  [unwired: 5 in]
      n62 = call "Keithley_ConfirmJump.vi"("VISA resource name in"=w305, "error in"=w304, "Gate Voltage\nInitial (V)"="Keithley #3 Vg Init. (V)") -> ("VISA resource name out"=w309:refnum<visa-resource-name>, "Voltage OK?"=w310:bool, "error out"=w308:errorcluster)  [unwired: 4 in, 1 out]
      n63 = case shown="True" w310 {
        tunnel: w309 -> [w348 w360]
        tunnel: w308 -> [w347 w359]
        tunnel: [w348 w353] -> w298
        tunnel: [w347 w354] -> w297
        tunnel: "Keithley #3 Vg Max (V)" -> [_ w358]
        tunnel: "Keithley #3 Vg Min (V)" -> [_ w357]
        tunnel: w290 -> [_ w352]
        tunnel: w289 -> [_ w351]
        tunnel: "Keithley #3 Vg Init. (V)" -> [_ w350]
        tunnel: "Keith#3 Comp. Lvl" -> [_ w349]
        frame False {
        }
        frame True {
          n64 = Absolute Value(x=w358) -> (abs(x)=w362:dbl)
          n65 = Absolute Value(x=w357) -> (abs(x)=w363:dbl)
          n66 = Max & Min(x=w362, y=w363) -> (max(x,y)=w367:dbl)  [unwired: 1 out]
          n67 = Format Into String(format string="%.;SOUR:VOLT:RANG %g ", w367) -> (resulting string=w366:string)  [unwired: 2 in, 1 out]
          n68 = call <instrlib>:"Enable Output.vi"("error in (no error)"=w359, "VISA resource name"=w360) -> ("error out"=w364:errorcluster, "VISA resource name out"=w365:refnum<visa-resource-name>)  [unwired: 8 in]
          n69 = VISA Write(VISA resource name=w365, write buffer=w366, error in (no error)=w364) -> (VISA resource name out=w356:refnum<visa-resource-name>, error out=w355:errorcluster)  [unwired: 1 out]
          n70 = call <instrlib>:"Configure Output.vi"("Output Type  (0: Immediate)"=w351, "Source Mode  (0: Voltage)"=w352, "error in (no error)"=w355, "Compliance  Level (0.1)"=w349, "Output Level (0)"=w350, "VISA resource name"=w356) -> ("error out"=w354:errorcluster, "VISA resource name out"=w353:refnum<visa-resource-name>)  [unwired: 4 in]
        }
      }
      n71 = call <instrlib>:"Configure Reference.vi"("VISA resource name"=w330, "Auto Phase (T: Enabled)"="SR830 #3 \nAuto Phase", "Manual Phase (0 Degree)"="SR830 #3 Manual \nPhase", "Reference Source (1: Internal)"="SR830 #3 Reference Source", "Sine Output Amplitude (1 V)"="SR830 #3 Sine \nOutput Amplitude", "Detection Harmonic Number (1)"="SR830 #3 Detection Harm. Num.", "error in (no error)"=w329, "Internal Reference Frequency (1000 Hz)"="SR830 #3 Internal \nReference Frequency") -> ("VISA resource name out"=w327:refnum<visa-resource-name>, "error out"=w328:errorcluster)  [unwired: 6 in]
      n72 = call <instrlib>:"Configure Filter.vi"("Enable Sync Filter (F: Disable)"="SR830 #3\nSync Filter", "error in (no error)"=w328, "Low Pass Filter Slope (1: 12dB/oct)"="SR830 #3 Low\nPass Filter Slope", "Time Constant (8: 100ms)"="SR830 #3 \nTime Constant", "VISA resource name"=w327) -> ("error out"=w313:errorcluster, "VISA resource name out"=w314:refnum<visa-resource-name>)  [unwired: 5 in]
      n73 = call <instrlib>:"Configure Sensitivity and Reserve.vi"("error in (no error)"=w313, "Sensitivity (-1: Auto gain)"="SR830 #3\nSensitivity", "Dynamic Reserve (-1: Auto Reserve)"="SR830 #3 \nDynamic Reserve", "VISA resource name"=w314) -> ("error out"=w295:errorcluster, "VISA resource name out"=w296:refnum<visa-resource-name>)  [unwired: 6 in]
      n74 = Bundle("VISA resource name out"=w298, "error out"=w297, "VISA resource name out"=w296, "error out"=w295, "Keithley #3 Vg Init. (V)"="Keithley #3 Vg Init. (V)", "Keithley #3 Vg Max (V)"="Keithley #3 Vg Max (V)", "Keithley #3 Vg Min (V)"="Keithley #3 Vg Min (V)", "Keithley #3 Vg Step (V)"="Keithley #3 Vg Step (V)", "Keith#3 Comp. Lvl"="Keith#3 Comp. Lvl") -> (w291:T13)  [unwired: 1 in]
    }
  }
  n75 = Concatenate Strings("<File Name>.txt (Don't add extension)", w98) -> (w104:string)
  n76 = Build Path(base path="Data Save Path:", name or relative path=w104) -> (appended path=w103:path)
  n77 = Concatenate Strings(w82, w70) -> (w69:string)
  n78 = call <vilib>:"Check if File or Folder Exists.vi"("path"=w103) -> ("file or folder exists?"=w102:bool, "dup path"=w101:path)  [unwired: 8 in, 1 out]
  n79 = case shown="True" w102 {
    tunnel: [w368 w369] -> w96
    tunnel: w101 -> [w368 _]
    tunnel: "Data Save Path:" -> [_ w370]
    tunnel: "<File Name>.txt (Don't add extension)" -> [_ w372]
    tunnel: w98 -> [_ w371]
    frame False {
    }
    frame True {
      n80 = while {
        tunnel: w372 -> [w375]
        tunnel: w371 -> [w380]
        tunnel: w370 -> [w378]
        tunnel: [w376] -> w369
        i -> [w382]
        stop <- w384 stop-if-true
        n81 = Concatenate Strings(w375, "_" ("string")) -> (w374:string)
        n82 = Format Into String(format string="%0.0f", initial string=w374, w382) -> (resulting string=w381:string)  [unwired: 1 in, 1 out]
        n83 = Concatenate Strings(w381, w380) -> (w379:string)
        n84 = Build Path(base path=w378, name or relative path=w379) -> (appended path=w377:path)
        n85 = call <vilib>:"Check if File or Folder Exists.vi"("path"=w377) -> ("file or folder exists?"=w385:bool, "dup path"=w376:path)  [unwired: 8 in, 1 out]
        n86 = Not(x=w385) -> (.not. x?=w384:bool)
      }
    }
  }
  "Actual Save Path" <- w96
  n87 = Concatenate Strings(w69, w68, w70) -> (w67:string)
  n88 = call-poly <instrlib>:"Signals (Read).vi"("ISOBUS address"="ISOBUS address 3", "Mercury Reference In"="Mercury Reference In") -> ()  [unwired: 5 in, 5 out]
  n89 = Unbundle By Name("Connection Details") -> ("IP Address"=w11:string, "VISA resource name"=w10:refnum<visa-resource-name>, "Comms Layer"=w9:T3, "Serial Configuration"=w13:T6, "ISOBUS address"=w12:T1)
  n90 = call-poly <instrlib>:"Configuration (Read).vi"("ISOBUS address"="ISOBUS address 2", "Mercury Reference In"="Mercury Reference In 2") -> ()  [unwired: 1 in, 9 out]
  n91 = Open/Create/Replace File(file path (use dialog)=w96, operation (0:open)=T8."create") -> (refnum out=w72:refnum<file>, error out=w71:errorcluster)  [unwired: 4 in, 1 out]
  n92 = Write to Text File(file (use dialog)=w72, text=w67, error in=w71) -> (refnum out=w46:refnum<file>, error out=w62:errorcluster)  [unwired: 1 in, 1 out]
  n93 = call-poly <instrlib>:"Signals (Read).vi"() -> ()  [unwired: 3 in, 9 out]
  n94 = call-poly <instrlib>:"Signals (Read).vi"() -> ()  [unwired: 3 in, 9 out]
  n95 = call-poly <instrlib>:"Signals (Read).vi"() -> ()  [unwired: 3 in, 9 out]
  n96 = call "OpenQDInstrument.vi"("Remote"="Remote", "IP Address"="127.0.0.1", "Instrument Type"=w95) -> ("error out"=w107:errorcluster, "Instrument Ref"=w106:refnum<k24>)  [unwired: 5 in]
  n97 = call-poly <instrlib>:"Open.vi"("IP Address"=w11, "error in (no error)"=errorcluster {"status"=FALSE, "code"=0, "source"=""}, "Serial Configuration"=w13, "Comms Layer"=w9, "VISA resource name"=w10) -> ("error out"=w15:errorcluster, "Mercury Reference Out"=w16:T2, "S/W Version(s)"=w7:string[])  [unwired: 2 in, 2 out]
  n98 = call "WaitFor.vi"("Wait For Chamber"=TRUE ("WaitForChamber"), "Wait For Position"=FALSE ("WaitForPosition"), "Wait For Field"=FALSE ("WaitForField"), "Wait For Temperature"=FALSE ("WaitForTemperature"), "error in (no error)"=w107, "Instrument Ref In"=w106) -> ("error out"=w111:errorcluster, "Instrument Ref Out"=w110:refnum<k24>)  [unwired: 4 in]
  n99 = call-poly <instrlib>:"Configuration (Read).vi"("ISOBUS address"=w12, "error in"=w15, "Mercury Reference In"=w16) -> ("Devices"=w5:string[])  [unwired: 8 out]
  n100 = call "GetChamber.vi"("error in (no error)"=w111, "Instrument Ref In"=w110) -> ("Chamber\nStatus"=→"Chamber Status":i32, "error out"=w64:errorcluster, "Instrument Ref Out"=w65:refnum<k24>)  [unwired: 2 in, 1 out]
  n101 = Bundle("Devices"=w5, "S/W Version(s)"=w7) -> (→"Device Details":T5)  [unwired: 1 out]
  n102 = Bundle("array"=w42, "array"=w42, "array"=w42, "array"=w42) -> (w45:T14)  [unwired: 1 in]
  n103 = Bundle("array"=w44, "array"=w44) -> (w43:cluster{"array":dbl[], "array":dbl[]})  [unwired: 1 in]
  n104 = while {
    shift-right: [w393] -> _
    shift-left: w66 -> [w395]
    shift-right: [w392] -> _
    shift-left: w66 -> [w394]
    shift-right: [w390] -> _
    shift-left: w66 -> [w391]
    shift-right: [w416] -> w60
    shift-left: w65 -> [w419]
    shift-right: [w414] -> w61
    shift-left: w64 -> [w418]
    shift-right: [w398] -> w59
    shift-left: w46 -> [w399]
    shift-right: [w396] -> w58
    shift-left: w62 -> [w397]
    shift-right: [w408] -> w41
    shift-left: w57 -> [w411]
    shift-right: [w407] -> w39
    shift-left: w56 -> [w410]
    shift-right: [w406] -> w40
    shift-left: w55 -> [w409]
    tunnel: w51 -> [w400]
    tunnel: [w400] -> w50
    shift-right: [w386] -> _
    shift-left: w45 -> [w389]
    shift-right: [w387] -> _
    shift-left: w43 -> [w388]
    stop <- "program_stop" stop-if-true
    n105 = flat-sequence {
      tunnel: w419 -> [w428]
      tunnel: w418 -> [w427]
      tunnel: [w426] -> w417
      tunnel: [w425] -> w415
      tunnel: [w422] -> w401
      tunnel: [w454] -> w413
      tunnel: w417 -> [w454]
      tunnel: [w453] -> w412
      tunnel: w415 -> [w453]
      tunnel: w411 -> [w452]
      tunnel: w410 -> [w451]
      tunnel: w409 -> [w450]
      tunnel: [w449] -> w408
      tunnel: [w448] -> w407
      tunnel: [w447] -> w406
      tunnel: w400 -> [w446]
      tunnel: [w442] -> w405
      tunnel: [w441] -> w404
      tunnel: [w440] -> w403
      tunnel: [w439] -> w402
      tunnel: w401 -> [w439]
      tunnel: w395 -> [w438]
      tunnel: w394 -> [w437]
      tunnel: [w436] -> w393
      tunnel: [w435] -> w392
      tunnel: w391 -> [w434]
      tunnel: [w433] -> w390
      tunnel: [w764] -> w416
      tunnel: w413 -> [w764]
      tunnel: [w763] -> w414
      tunnel: w412 -> [w763]
      tunnel: w405 -> [w760]
      tunnel: w404 -> [w758]
      tunnel: w403 -> [w757]
      tunnel: w402 -> [w759]
      tunnel: w400 -> [w762]
      tunnel: w399 -> [w744]
      tunnel: w397 -> [w742]
      tunnel: [w743] -> w398
      tunnel: [w741] -> w396
      tunnel: w389 -> [w730]
      tunnel: w388 -> [w736]
      tunnel: [w735] -> w387
      tunnel: [w729] -> w386
      frame #0 {
        # "Oxford Temp & Field"
        n106 = call "GetTemperature.vi"("error in (no error)"=w427, "Instrument Ref In"=w428) -> ("Temperature"=w424:dbl, "error out"=w431:errorcluster, "Instrument Ref Out"=w432:refnum<k24>)  [unwired: 3 in, 2 out]
        "Temperature" <- w424
        n107 = local write "Measuring"(TRUE ("Measuring")) -> ()
        n108 = Wait (ms)(milliseconds to wait=u32 200) -> ()  [unwired: 1 out]
        n109 = call "GetField.vi"("error in (no error)"=w431, "Instrument Ref In"=w432) -> ("Field"=w423:dbl, "error out"=w425:errorcluster, "Instrument Ref Out"=w426:refnum<k24>)  [unwired: 3 in, 2 out]
        "Field" <- w423
        n110 = Bundle("Temperature"=w424, "Field"=w423) -> (w422:cluster{"Temperature":dbl, "Field":dbl})  [unwired: 1 in]
      }
      frame #1 {
        # "Keith & SRs"
        n111 = Unbundle(w446) -> ("System #1 Enabled/Disabled"=w445:bool, "System #2 Enabled/Disabled"=w444:bool, "System #3 Enabled/Disabled"=w443:bool)
        n112 = stacked-sequence {
          tunnel: w452 -> [w460 _ _]
          tunnel: w451 -> [_ w541 _]
          tunnel: w450 -> [_ _ w623]
          tunnel: [w459 _ _] -> w449
          tunnel: [_ w542 _] -> w448
          tunnel: [_ _ w624] -> w447
          tunnel: w445 -> [w458 _ _]
          tunnel: w444 -> [_ w540 _]
          tunnel: w443 -> [_ _ w622]
          tunnel: [w457 _ _] -> w442
          tunnel: [_ w539 _] -> w441
          tunnel: [_ _ w621] -> w440
          tunnel: w438 -> [w456 _ _]
          tunnel: w437 -> [_ w538 _]
          tunnel: [w455 _ _] -> w436
          tunnel: [_ w537 _] -> w435
          tunnel: w434 -> [_ _ w620]
          tunnel: [_ _ w619] -> w433
          frame #0 {
            # "Keithley & SR #1"
            n113 = case shown="True" w458 {
              tunnel: w460 -> [w463 w466]
              tunnel: [w463 w481] -> w459
              tunnel: [T15 {"Voltage"=0.0, "Current"=0.0, "X-Value"=0.0, "R-Value"=0.0, "Theta-Value"=0.0} w467] -> w457
              tunnel: w456 -> [w461 w465]
              tunnel: [w461 w464] -> w455
              frame False {
              }
              frame True {
                n114 = Unbundle(w466) -> ("VISA resource name out"=w478:refnum<visa-resource-name>, "error out"=w477:errorcluster, "VISA resource name out"=w480:refnum<visa-resource-name>, "error out"=w479:errorcluster)  [unwired: 5 out]
                n115 = flat-sequence {
                  tunnel: [w494] -> w474
                  tunnel: [w493] -> w473
                  tunnel: [w491] -> w470
                  tunnel: [w490] -> w469
                  tunnel: [w489] -> w468
                  tunnel: w480 -> [w488]
                  tunnel: w479 -> [w487]
                  tunnel: [w500] -> w486
                  tunnel: [w499] -> w485
                  tunnel: [w495] -> w484
                  tunnel: [w498] -> w471
                  tunnel: w478 -> [w497]
                  tunnel: w477 -> [w496]
                  tunnel: [w495] -> w472
                  tunnel: w486 -> [w509]
                  tunnel: w485 -> [w508]
                  tunnel: [w507] -> w475
                  tunnel: w484 -> [w506]
                  tunnel: [w510] -> w483
                  tunnel: [w505] -> w482
                  tunnel: [w504] -> w476
                  tunnel: w466 -> [w502]
                  tunnel: w465 -> [w501]
                  tunnel: [w531] -> w464
                  tunnel: w483 -> [w532]
                  tunnel: w482 -> [w530]
                  frame #0 {
                    n116 = call-poly <instrlib>:"Read.vi"("error in (no error)"=w487, "VISA resource name"=w488) -> ("error out"=w493:errorcluster, "Parameter Values"=w492:T17, "VISA resource name out"=w494:refnum<visa-resource-name>)  [unwired: 7 in]
                    n117 = Unbundle(w492) -> ("X-Value"=w491:dbl, "R-Value"=w490:dbl, "Theta-Value"=w489:dbl)  [unwired: 8 out]
                    "X-Value" <- w491
                    "Theta-Value" <- w489
                    "R-Value" <- w490
                  }
                  frame #1 {
                    n118 = call-poly <instrlib>:"Read.vi"("VISA resource name"=w497, "error in (no error)"=w496) -> ("Voltage"=w495:sgl, "VISA resource name out"=w500:refnum<visa-resource-name>, "Current"=w498:sgl, "error out"=w499:errorcluster)  [unwired: 7 in, 3 out]
                    "Voltage #1" <- w495
                    "Leakage Current #1" <- w498
                  }
                  frame #2 {
                    n119 = local read "Keithley #1 Ramp"() -> (w503:bool)
                    n120 = case shown="True" w503 {
                      tunnel: [w512 w529] -> w510
                      tunnel: w509 -> [w514 w528]
                      tunnel: w508 -> [w513 w527]
                      tunnel: [w513 w526] -> w507
                      tunnel: [w514 w525] -> w504
                      tunnel: w506 -> [_ w524]
                      tunnel: [FALSE ("END?") w523] -> w505
                      tunnel: w502 -> [_ w521]
                      tunnel: w501 -> [w512 w515]
                      frame False {
                      }
                      frame True {
                        n121 = Unbundle(w521) -> ("Keithley #1 Vg Init. (V)"=w520:dbl, "Keithley #1 Vg Max (V)"=w519:dbl, "Keithley #1 Vg Min (V)"=w518:dbl, "Keithley #1 Vg Step (V)"=w517:dbl, "Keith#1 Comp. Lvl"=w516:dbl)  [unwired: 4 out]
                        n122 = call "Keithley_Iterator.vi"("VISA resource name"=w528, "High Voltage"=w519, "Low Voltage"=w518, "Initial Voltage"=w520, "Iteration Input"=w515, "Current Voltage"=w524, "error in (no error)"=w527, "Voltage Step"=w517, "Compliance  Level (0.1)"=w516) -> ("VISA resource name out"=w525:refnum<visa-resource-name>, "Iteration Output"=w529:i32, "END?"=w523:bool, "error out"=w526:errorcluster)  [unwired: 2 in, 1 out]
                        n123 = property on="Keithley #1 Ramp" class="Bool (strict)"("DisabledEnum"=T16."Disabled and Grayed Out" ("Disabled")) -> ()  [unwired: 2 in, 2 out]
                      }
                    }
                  }
                  frame #3 {
                    n124 = case shown="True" w530 {
                      tunnel: w532 -> [w533 _]
                      tunnel: [w533 0 ("Iteration Output")] -> w531
                      frame False {
                      }
                      frame True {
                        # "Reset Iterator"
                        n125 = local write "Keithley #1 Ramp"(FALSE ("Keithley #1 Ramp")) -> ()
                        n126 = property on="Keithley #1 Ramp" class="Bool (strict)"("DisabledEnum"=T16."Enabled" ("Disabled")) -> ()  [unwired: 2 in, 2 out]
                      }
                    }
                  }
                }
                n127 = Bundle("Voltage"=w472, "Current"=w471, "X-Value"=w470, "R-Value"=w469, "Theta-Value"=w468) -> (w467:T15)  [unwired: 1 in]
                n128 = Bundle(cluster=w466, "VISA resource name out"=w476, "error out"=w475, "VISA resource name out"=w474, "error out"=w473) -> (w481:T10)  [unwired: 5 in]
              }
            }
          }
          frame #1 {
            # "Keithley & SR #2"
            n129 = case shown="True" w540 {
              tunnel: [w545 w563] -> w542
              tunnel: w541 -> [w545 w547]
              tunnel: [T15 {"Voltage"=0.0, "Current"=0.0, "X-Value"=0.0, "R-Value"=0.0, "Theta-Value"=0.0} w549] -> w539
              tunnel: w538 -> [w543 w548]
              tunnel: [w543 w546] -> w537
              frame False {
              }
              frame True {
                n130 = Unbundle(w547) -> ("VISA resource name out"=w556:refnum<visa-resource-name>, "error out"=w555:errorcluster, "VISA resource name out"=w558:refnum<visa-resource-name>, "error out"=w557:errorcluster)  [unwired: 5 out]
                n131 = flat-sequence {
                  tunnel: [w576] -> w562
                  tunnel: [w575] -> w561
                  tunnel: [w573] -> w552
                  tunnel: [w572] -> w551
                  tunnel: [w571] -> w550
                  tunnel: w558 -> [w570]
                  tunnel: w557 -> [w569]
                  tunnel: [w582] -> w568
                  tunnel: [w581] -> w567
                  tunnel: [w579] -> w566
                  tunnel: [w580] -> w553
                  tunnel: [w579] -> w554
                  tunnel: w556 -> [w578]
                  tunnel: w555 -> [w577]
                  tunnel: w568 -> [w591]
                  tunnel: w567 -> [w590]
                  tunnel: [w589] -> w559
                  tunnel: [w588] -> w560
                  tunnel: w566 -> [w587]
                  tunnel: [w592] -> w565
                  tunnel: [w586] -> w564
                  tunnel: w548 -> [w584]
                  tunnel: w547 -> [w583]
                  tunnel: [w613] -> w546
                  tunnel: w565 -> [w614]
                  tunnel: w564 -> [w612]
                  frame #0 {
                    n132 = call-poly <instrlib>:"Read.vi"("error in (no error)"=w569, "VISA resource name"=w570) -> ("error out"=w575:errorcluster, "Parameter Values"=w574:T17, "VISA resource name out"=w576:refnum<visa-resource-name>)  [unwired: 7 in]
                    n133 = Unbundle(w574) -> ("X-Value"=w573:dbl, "R-Value"=w572:dbl, "Theta-Value"=w571:dbl)  [unwired: 8 out]
                    "X-Value 2" <- w573
                    "Theta-Value 2" <- w571
                    "R-Value 2" <- w572
                  }
                  frame #1 {
                    n134 = call-poly <instrlib>:"Read.vi"("VISA resource name"=w578, "error in (no error)"=w577) -> ("Voltage"=w579:sgl, "VISA resource name out"=w582:refnum<visa-resource-name>, "Current"=w580:sgl, "error out"=w581:errorcluster)  [unwired: 7 in, 3 out]
                    "Voltage #2" <- w579
                    "Leakage Current #2" <- w580
                  }
                  frame #2 {
                    n135 = local read "Keithley #2 Ramp"() -> (w585:bool)
                    n136 = case shown="True" w585 {
                      tunnel: [w594 w611] -> w592
                      tunnel: w591 -> [w596 w610]
                      tunnel: w590 -> [w595 w609]
                      tunnel: [w595 w608] -> w589
                      tunnel: [w596 w607] -> w588
                      tunnel: w587 -> [_ w606]
                      tunnel: [FALSE ("END?") w605] -> w586
                      tunnel: w584 -> [w594 w603]
                      tunnel: w583 -> [_ w602]
                      frame False {
                      }
                      frame True {
                        n137 = Unbundle(w602) -> ("Keithley #2 Vg Init. (V)"=w601:dbl, "Keithley #2 Vg Max (V)"=w600:dbl, "Keithley #2 Vg Min (V)"=w599:dbl, "Keithley #2 Vg Step (V)"=w598:dbl, "Keith#2 Comp. Lvl"=w597:dbl)  [unwired: 4 out]
                        n138 = call "Keithley_Iterator.vi"("VISA resource name"=w610, "High Voltage"=w600, "Low Voltage"=w599, "Initial Voltage"=w601, "Iteration Input"=w603, "Current Voltage"=w606, "error in (no error)"=w609, "Voltage Step"=w598, "Compliance  Level (0.1)"=w597) -> ("VISA resource name out"=w607:refnum<visa-resource-name>, "Iteration Output"=w611:i32, "END?"=w605:bool, "error out"=w608:errorcluster)  [unwired: 2 in, 1 out]
                        n139 = property on="Keithley #2 Ramp" class="Bool (strict)"("DisabledEnum"=T16."Disabled and Grayed Out" ("Disabled")) -> ()  [unwired: 2 in, 2 out]
                      }
                    }
                  }
                  frame #3 {
                    n140 = case shown="True" w612 {
                      tunnel: w614 -> [w615 _]
                      tunnel: [w615 0 ("Iteration Output")] -> w613
                      frame False {
                      }
                      frame True {
                        # "Reset Iterator"
                        n141 = local write "Keithley #2 Ramp"(FALSE ("Keithley #1 Ramp")) -> ()
                        n142 = property on="Keithley #2 Ramp" class="Bool (strict)"("DisabledEnum"=T16."Enabled" ("Disabled")) -> ()  [unwired: 2 in, 2 out]
                      }
                    }
                  }
                }
                n143 = Bundle("Voltage"=w554, "Current"=w553, "X-Value"=w552, "R-Value"=w551, "Theta-Value"=w550) -> (w549:T15)  [unwired: 1 in]
                n144 = Bundle(cluster=w547, "VISA resource name out"=w560, "error out"=w559, "VISA resource name out"=w562, "error out"=w561) -> (w563:T12)  [unwired: 5 in]
              }
            }
          }
          frame #2 {
            # "Keithley & SR #3"
            n145 = case shown="True" w622 {
              tunnel: [w627 w645] -> w624
              tunnel: w623 -> [w627 w630]
              tunnel: [T15 {"Voltage"=0.0, "Current"=0.0, "X-Value"=0.0, "R-Value"=0.0, "Theta-Value"=0.0} w631] -> w621
              tunnel: w620 -> [w625 w629]
              tunnel: [w625 w628] -> w619
              frame False {
              }
              frame True {
                n146 = Unbundle(w630) -> ("VISA resource name out"=w644:refnum<visa-resource-name>, "error out"=w643:errorcluster, "VISA resource name out"=w642:refnum<visa-resource-name>, "error out"=w641:errorcluster)  [unwired: 5 out]
                n147 = flat-sequence {
                  tunnel: [w658] -> w640
                  tunnel: [w657] -> w639
                  tunnel: [w655] -> w634
                  tunnel: [w654] -> w633
                  tunnel: [w653] -> w632
                  tunnel: w642 -> [w652]
                  tunnel: w641 -> [w651]
                  tunnel: [w664] -> w650
                  tunnel: [w663] -> w649
                  tunnel: [w661] -> w648
                  tunnel: [w662] -> w635
                  tunnel: [w661] -> w636
                  tunnel: w644 -> [w660]
                  tunnel: w643 -> [w659]
                  tunnel: w650 -> [w673]
                  tunnel: w649 -> [w672]
                  tunnel: [w671] -> w637
                  tunnel: [w670] -> w638
                  tunnel: w648 -> [w669]
                  tunnel: [w674] -> w647
                  tunnel: [w668] -> w646
                  tunnel: w630 -> [w666]
                  tunnel: w629 -> [w665]
                  tunnel: [w695] -> w628
                  tunnel: w647 -> [w696]
                  tunnel: w646 -> [w694]
                  frame #0 {
                    n148 = call-poly <instrlib>:"Read.vi"("error in (no error)"=w651, "VISA resource name"=w652) -> ("error out"=w657:errorcluster, "Parameter Values"=w656:T17, "VISA resource name out"=w658:refnum<visa-resource-name>)  [unwired: 7 in]
                    n149 = Unbundle(w656) -> ("X-Value"=w655:dbl, "R-Value"=w654:dbl, "Theta-Value"=w653:dbl)  [unwired: 8 out]
                    "X-Value 3" <- w655
                    "Theta-Value 3" <- w653
                    "R-Value 3" <- w654
                  }
                  frame #1 {
                    n150 = call-poly <instrlib>:"Read.vi"("VISA resource name"=w660, "error in (no error)"=w659) -> ("Voltage"=w661:sgl, "VISA resource name out"=w664:refnum<visa-resource-name>, "Current"=w662:sgl, "error out"=w663:errorcluster)  [unwired: 7 in, 3 out]
                    "Voltage #3" <- w661
                    "Leakage Current #3" <- w662
                  }
                  frame #2 {
                    n151 = local read "Keithley #3 Ramp"() -> (w667:bool)
                    n152 = case shown="True" w667 {
                      tunnel: [w676 w693] -> w674
                      tunnel: w673 -> [w678 w692]
                      tunnel: w672 -> [w677 w691]
                      tunnel: [w677 w690] -> w671
                      tunnel: [w678 w689] -> w670
                      tunnel: w669 -> [_ w688]
                      tunnel: [FALSE ("END?") w687] -> w668
                      tunnel: w666 -> [_ w685]
                      tunnel: w665 -> [w676 w684]
                      frame False {
                      }
                      frame True {
                        n153 = Unbundle(w685) -> ("Keithley #3 Vg Init. (V)"=w683:dbl, "Keithley #3 Vg Max (V)"=w682:dbl, "Keithley #3 Vg Min (V)"=w681:dbl, "Keithley #3 Vg Step (V)"=w680:dbl, "Keith#3 Comp. Lvl"=w679:dbl)  [unwired: 4 out]
                        n154 = call "Keithley_Iterator.vi"("VISA resource name"=w692, "High Voltage"=w682, "Low Voltage"=w681, "Initial Voltage"=w683, "Iteration Input"=w684, "Current Voltage"=w688, "error in (no error)"=w691, "Voltage Step"=w680, "Compliance  Level (0.1)"=w679) -> ("VISA resource name out"=w689:refnum<visa-resource-name>, "Iteration Output"=w693:i32, "END?"=w687:bool, "error out"=w690:errorcluster)  [unwired: 2 in, 1 out]
                        n155 = property on="Keithley #3 Ramp" class="Bool (strict)"("DisabledEnum"=T16."Disabled and Grayed Out" ("Disabled")) -> ()  [unwired: 2 in, 2 out]
                      }
                    }
                  }
                  frame #3 {
                    n156 = case shown="True" w694 {
                      tunnel: w696 -> [w697 _]
                      tunnel: [w697 0 ("Iteration Output")] -> w695
                      frame False {
                      }
                      frame True {
                        # "Reset Iterator"
                        n157 = local write "Keithley #3 Ramp"(FALSE ("Keithley #1 Ramp")) -> ()
                        n158 = property on="Keithley #3 Ramp" class="Bool (strict)"("DisabledEnum"=T16."Enabled" ("Disabled")) -> ()  [unwired: 2 in, 2 out]
                      }
                    }
                  }
                }
                n159 = Bundle("Voltage"=w636, "Current"=w635, "X-Value"=w634, "R-Value"=w633, "Theta-Value"=w632) -> (w631:T15)  [unwired: 1 in]
                n160 = Bundle(cluster=w630, "VISA resource name out"=w638, "error out"=w637, "VISA resource name out"=w640, "error out"=w639) -> (w645:T13)  [unwired: 5 in]
              }
            }
          }
        }
      }
      frame #2 {
        w754 = "%.12f" ("format string")
        w751 = "\t"
        # "Theta"
        # "X"
        # "Current"
        # "Voltage"
        # "Field"
        # "Temperature"
        # "Write #3"
        # "Write #2"
        # "Write #1"
        # "Conclusion"
        n161 = Unbundle(w762) -> ("System #1 Enabled/Disabled"=w761:bool, "System #2 Enabled/Disabled"=w756:bool, "System #3 Enabled/Disabled"=w755:bool)
        n162 = Unbundle(w759) -> ("Temperature"=w739:dbl, "Field"=w737:dbl)
        n163 = local write "Measuring"(FALSE ("Measuring")) -> ()
        n164 = Format Into String(format string=w754, w739) -> (resulting string=w753:string)  [unwired: 2 in, 1 out]
        n165 = Format Into String(format string=w754, w737) -> (resulting string=w752:string)  [unwired: 2 in, 1 out]
        n166 = Concatenate Strings(w753, w751, w752) -> (w750:string)
        n167 = case shown="True" w761 {
          tunnel: w760 -> [_ w857]
          tunnel: w754 -> [_ w855]
          tunnel: w751 -> [_ w846]
          tunnel: w750 -> [w836 w847]
          tunnel: [w836 w848] -> w749
          tunnel: dbl[] [] ("array") -> [w835 w841]
          tunnel: [w835 w840] -> w727
          tunnel: [w835 w839] -> w726
          tunnel: [w835 w838] -> w725
          tunnel: [w835 w837] -> w724
          frame False {
          }
          frame True {
            n168 = Unbundle(w857) -> ("Voltage"=w845:sgl, "Current"=w844:sgl, "X-Value"=w843:dbl, "R-Value"=w856:dbl, "Theta-Value"=w842:dbl)
            n169 = Format Into String(format string=w855, w845) -> (resulting string=w854:string)  [unwired: 2 in, 1 out]
            n170 = Format Into String(format string=w855, w844) -> (resulting string=w853:string)  [unwired: 2 in, 1 out]
            n171 = Format Into String(format string=w855, w843) -> (resulting string=w852:string)  [unwired: 2 in, 1 out]
            n172 = Format Into String(format string=w855, w842) -> (resulting string=w850:string)  [unwired: 2 in, 1 out]
            n173 = Insert Into Array(array=w841, new element=w844) -> (w839:dbl[])  [unwired: 1 in]
            n174 = Insert Into Array(array=w841, new element=w845) -> (w840:dbl[])  [unwired: 1 in]
            n175 = Insert Into Array(array=w841, new element=w842) -> (w837:dbl[])  [unwired: 1 in]
            n176 = Insert Into Array(array=w841, new element=w843) -> (w838:dbl[])  [unwired: 1 in]
            n177 = Format Into String(format string=w855, initial string=w852, w856) -> (resulting string=w851:string)  [unwired: 1 in, 1 out]
            n178 = Concatenate Strings(w854, w846, w853, w846, w852, w846, w851, w846, w850) -> (w849:string)
            n179 = Concatenate Strings(w847, w846, w849) -> (w848:string)
          }
        }
        n180 = Unbundle(w736) -> ("array"=w740:dbl[], "array"=w738:dbl[])
        n181 = case shown="True" w756 {
          tunnel: w758 -> [_ w834]
          tunnel: w754 -> [_ w832]
          tunnel: w751 -> [_ w825]
          tunnel: w749 -> [w810 w826]
          tunnel: [w810 w823] -> w748
          tunnel: w727 -> [w809 w822]
          tunnel: w726 -> [w808 w821]
          tunnel: w725 -> [w807 w820]
          tunnel: w724 -> [w806 w819]
          tunnel: [w809 w814] -> w723
          tunnel: [w808 w813] -> w722
          tunnel: [w807 w812] -> w721
          tunnel: [w806 w811] -> w720
          frame False {
          }
          frame True {
            n182 = Unbundle(w834) -> ("Voltage"=w818:sgl, "Current"=w817:sgl, "X-Value"=w816:dbl, "R-Value"=w833:dbl, "Theta-Value"=w815:dbl)
            n183 = Format Into String(format string=w832, w818) -> (resulting string=w831:string)  [unwired: 2 in, 1 out]
            n184 = Format Into String(format string=w832, w817) -> (resulting string=w830:string)  [unwired: 2 in, 1 out]
            n185 = Format Into String(format string=w832, w816) -> (resulting string=w829:string)  [unwired: 2 in, 1 out]
            n186 = Format Into String(format string=w832, w815) -> (resulting string=w827:string)  [unwired: 2 in, 1 out]
            n187 = Insert Into Array(array=w821, new element=w817) -> (w813:dbl[])  [unwired: 1 in]
            n188 = Insert Into Array(array=w822, new element=w818) -> (w814:dbl[])  [unwired: 1 in]
            n189 = Insert Into Array(array=w819, new element=w815) -> (w811:dbl[])  [unwired: 1 in]
            n190 = Insert Into Array(array=w820, new element=w816) -> (w812:dbl[])  [unwired: 1 in]
            n191 = Format Into String(format string=w832, initial string=w829, w833) -> (resulting string=w828:string)  [unwired: 1 in, 1 out]
            n192 = Concatenate Strings(w831, w825, w830, w825, w829, w825, w828, w825, w827) -> (w824:string)
            n193 = Concatenate Strings(w826, w825, w824) -> (w823:string)
          }
        }
        n194 = case shown="True" w755 {
          tunnel: w757 -> [_ w805]
          tunnel: w754 -> [_ w803]
          tunnel: w751 -> [_ w796]
          tunnel: w748 -> [w781 w795]
          tunnel: [w781 w794] -> w747
          tunnel: w723 -> [w780 w793]
          tunnel: w722 -> [w779 w792]
          tunnel: w721 -> [w778 w791]
          tunnel: w720 -> [w777 w790]
          tunnel: [w780 w785] -> w719
          tunnel: [w779 w784] -> w718
          tunnel: [w778 w783] -> w717
          tunnel: [w777 w782] -> w716
          frame False {
          }
          frame True {
            n195 = Unbundle(w805) -> ("Voltage"=w789:sgl, "Current"=w788:sgl, "X-Value"=w787:dbl, "R-Value"=w804:dbl, "Theta-Value"=w786:dbl)
            n196 = Format Into String(format string=w803, w789) -> (resulting string=w802:string)  [unwired: 2 in, 1 out]
            n197 = Format Into String(format string=w803, w788) -> (resulting string=w801:string)  [unwired: 2 in, 1 out]
            n198 = Format Into String(format string=w803, w787) -> (resulting string=w800:string)  [unwired: 2 in, 1 out]
            n199 = Format Into String(format string=w803, w786) -> (resulting string=w798:string)  [unwired: 2 in, 1 out]
            n200 = Insert Into Array(array=w792, new element=w788) -> (w784:dbl[])  [unwired: 1 in]
            n201 = Insert Into Array(array=w793, new element=w789) -> (w785:dbl[])  [unwired: 1 in]
            n202 = Insert Into Array(array=w790, new element=w786) -> (w782:dbl[])  [unwired: 1 in]
            n203 = Insert Into Array(array=w791, new element=w787) -> (w783:dbl[])  [unwired: 1 in]
            n204 = Format Into String(format string=w803, initial string=w800, w804) -> (resulting string=w799:string)  [unwired: 1 in, 1 out]
            n205 = Concatenate Strings(w802, w796, w801, w796, w800, w796, w799, w796, w798) -> (w797:string)
            n206 = Concatenate Strings(w795, w796, w797) -> (w794:string)
          }
        }
        n207 = Unbundle(w730) -> ("array"=w731:dbl[][], "array"=w732:dbl[][], "array"=w733:dbl[][], "array"=w734:dbl[][])
        n208 = Build Array (concatenate)(w732, w718) -> (w714:dbl[][])
        n209 = Build Array (concatenate)(w731, w719) -> (w715:dbl[][])
        n210 = Build Array (concatenate)(w734, w716) -> (w712:dbl[][])
        n211 = Build Array (concatenate)(w733, w717) -> (w713:dbl[][])
        n212 = Concatenate Strings(w747, "\r\n") -> (w745:string)
        n213 = Transpose 2D Array(2D array=w714) -> (transposed array=w710:dbl[][])
        n214 = Transpose 2D Array(2D array=w715) -> (transposed array=w711:dbl[][])
        n215 = Transpose 2D Array(2D array=w712) -> (transposed array=w706:dbl[][])
        n216 = Bundle(w715, w714, w713, w712) -> (w729:cluster{dbl[][], dbl[][], dbl[][], dbl[][]})  [unwired: 1 in]
        n217 = Transpose 2D Array(2D array=w713) -> (transposed array=w708:dbl[][])
        n218 = Build Array (concatenate)(w738, w737) -> (w703:dbl[])
        n219 = Build Array (concatenate)(w740, w739) -> (w704:dbl[])
        n220 = Write to Text File(file (use dialog)=w744, text=w745, error in=w742) -> (refnum out=w743:refnum<file>, error out=w741:errorcluster)  [unwired: 1 in, 1 out]
        n221 = for {
          tunnel: w711 -> [w772] mode=indexing
          tunnel: w710 -> [w776] mode=indexing
          tunnel: [w775] -> w709 mode=indexing
          tunnel: w708 -> [w768] mode=indexing
          tunnel: [w774] -> w707 mode=indexing
          tunnel: w706 -> [w773] mode=indexing
          tunnel: [w771] -> w705 mode=indexing
          tunnel: w704 -> [w770]
          tunnel: w703 -> [w769]
          tunnel: [w767] -> w702 mode=indexing
          tunnel: [w766] -> w701 mode=indexing
          n222 = Bundle(w772, w776) -> (w775:cluster{dbl[], dbl[]})  [unwired: 1 in]
          n223 = Bundle(w772, w768) -> (w774:cluster{dbl[], dbl[]})  [unwired: 1 in]
          n224 = Bundle(w772, w773) -> (w771:cluster{dbl[], dbl[]})  [unwired: 1 in]
          n225 = Bundle(w769, w768) -> (w767:cluster{dbl[], dbl[]})  [unwired: 1 in]
          n226 = Bundle(w770, w768) -> (w766:cluster{dbl[], dbl[]})  [unwired: 1 in]
        }
        "Signal-T" <- w701
        "Leak-Vg" <- w709
        "Phase-Vg" <- w705
        "Signal-B" <- w702
        "Signal-Vg" <- w707
        n227 = Bundle(w704, w703) -> (w735:cluster{dbl[], dbl[]})  [unwired: 1 in]
      }
    }
    n228 = Wait (ms)(milliseconds to wait=u32 1000) -> ()  [unwired: 1 out]
  }
  n229 = call-poly <instrlib>:"Signals (Read).vi"() -> ()  [unwired: 3 in, 9 out]
  n230 = Close File(refnum=w59, error in=w58) -> (error out=w63:errorcluster)  [unwired: 1 out]
  n231 = call <vilib>:"Simple Error Handler.vi"("error in (no error)"=w63) -> ()  [unwired: 4 in, 5 out]
  n232 = Close Reference(reference=w60, error in (no error)=w61) -> ()  [unwired: 1 out]
  n233 = Unbundle(w50) -> ("System #1 Enabled/Disabled"=w49:bool, "System #2 Enabled/Disabled"=w48:bool, "System #3 Enabled/Disabled"=w47:bool)
  n234 = case shown="True" w48 {
    tunnel: w40 -> [_ w862]
    frame False {
    }
    frame True {
      n235 = Unbundle(w862) -> ("VISA resource name out"=w859:refnum<visa-resource-name>, "error out"=w858:errorcluster, "VISA resource name out"=w861:refnum<visa-resource-name>, "error out"=w860:errorcluster)  [unwired: 5 out]
      n236 = call <instrlib>:"Close.vi"("error in (no error)"=w860, "VISA resource name"=w861) -> ("error out"=w863:errorcluster)  [unwired: 9 in]
      n237 = call <instrlib>:"Close.vi"("error in (no error)"=w858, "VISA resource name"=w859) -> ("error out"=w864:errorcluster)  [unwired: 9 in]
      n238 = call <vilib>:"Simple Error Handler.vi"("error in (no error)"=w863) -> ()  [unwired: 4 in, 5 out]
      n239 = call <vilib>:"Simple Error Handler.vi"("error in (no error)"=w864) -> ()  [unwired: 4 in, 5 out]
    }
  }
  n240 = case shown="True" w49 {
    tunnel: w41 -> [_ w869]
    frame False {
    }
    frame True {
      n241 = Unbundle(w869) -> ("VISA resource name out"=w868:refnum<visa-resource-name>, "error out"=w867:errorcluster, "VISA resource name out"=w866:refnum<visa-resource-name>, "error out"=w865:errorcluster)  [unwired: 5 out]
      n242 = call <instrlib>:"Close.vi"("error in (no error)"=w865, "VISA resource name"=w866) -> ("error out"=w870:errorcluster)  [unwired: 9 in]
      n243 = call <instrlib>:"Close.vi"("error in (no error)"=w867, "VISA resource name"=w868) -> ("error out"=w871:errorcluster)  [unwired: 9 in]
      n244 = call <vilib>:"Simple Error Handler.vi"("error in (no error)"=w870) -> ()  [unwired: 4 in, 5 out]
      n245 = call <vilib>:"Simple Error Handler.vi"("error in (no error)"=w871) -> ()  [unwired: 4 in, 5 out]
    }
  }
  n246 = case shown="True" w47 {
    tunnel: w39 -> [_ w876]
    frame False {
    }
    frame True {
      n247 = Unbundle(w876) -> ("VISA resource name out"=w875:refnum<visa-resource-name>, "error out"=w874:errorcluster, "VISA resource name out"=w873:refnum<visa-resource-name>, "error out"=w872:errorcluster)  [unwired: 5 out]
      n248 = call <instrlib>:"Close.vi"("error in (no error)"=w872, "VISA resource name"=w873) -> ("error out"=w877:errorcluster)  [unwired: 9 in]
      n249 = call <instrlib>:"Close.vi"("error in (no error)"=w874, "VISA resource name"=w875) -> ("error out"=w878:errorcluster)  [unwired: 9 in]
      n250 = call <vilib>:"Simple Error Handler.vi"("error in (no error)"=w877) -> ()  [unwired: 4 in, 5 out]
      n251 = call <vilib>:"Simple Error Handler.vi"("error in (no error)"=w878) -> ()  [unwired: 4 in, 5 out]
    }
  }
  "Measuring" <- FALSE ("Measuring")
